vi "Calibration.vi"(7 "Show Front Panel":bool=TRUE, 8 "error in (no error)":errorcluster, 11 "Calibration File Path":path=path "C:/Program Files/GE/Dryer Performance Test/CalibrationDates.txt") -> (0 "error out":errorcluster, 3 "Calibration Data":string[][](array[string]))   [LabVIEW 2018]
uses:
  Type Definitions/Calibration.ctl
  Type Definitions/Calibration Time.ctl
  Type Definitions/Calibration SN.ctl
  Calibration Equipment.vi
  <vilib>/Utility/file.llb/Write Delimited Spreadsheet (string).vi
panel:
  out "concatenated string":string
  in  "Size":i32
  out "snta":string[](array[string])
  in  "Tab Control":enum32{"Calibration Dates", "Export Data"}(tab)
  in  "Equipment Description":T1
  in  "Manufacturer":T1
  in  "Model Number":T1
  in  "Calibration ID":T1
  in  "Complete":bool
  in  "Serial Number":T2
  in  "Last Calibrated":T3 {"Eq20" format="%<%x>T"; "Eq19" format="%<%x>T"; "Eq18" format="%<%x>T"; "Eq17" format="%<%x>T"; "Eq16" format="%<%x>T"; "Eq15" format="%<%x>T"; "Eq14" format="%<%x>T"; "Eq13" format="%<%x>T"; "Eq12" format="%<%x>T"; "Eq11" format="%<%x>T"; "Eq10" format="%<%x>T"; "Eq9" format="%<%x>T"; "Eq8" format="%<%x>T"; "Eq7" format="%<%x>T"; "Eq6" format="%<%x>T"; "Eq5" format="%<%x>T"; "Eq4" format="%<%x>T"; "Eq3" format="%<%x>T"; "Eq2" format="%<%x>T"; "Eq1" format="%<%x>T"}
  in  "Calibration Due":T3 {"Eq20" format="%<%x>T"; "Eq19" format="%<%x>T"; "Eq18" format="%<%x>T"; "Eq17" format="%<%x>T"; "Eq16" format="%<%x>T"; "Eq15" format="%<%x>T"; "Eq14" format="%<%x>T"; "Eq13" format="%<%x>T"; "Eq12" format="%<%x>T"; "Eq11" format="%<%x>T"; "Eq10" format="%<%x>T"; "Eq9" format="%<%x>T"; "Eq8" format="%<%x>T"; "Eq7" format="%<%x>T"; "Eq6" format="%<%x>T"; "Eq5" format="%<%x>T"; "Eq4" format="%<%x>T"; "Eq3" format="%<%x>T"; "Eq2" format="%<%x>T"; "Eq1" format="%<%x>T"}
  in  "Update":bool
  # "To Export Data: Right Click -> Export"
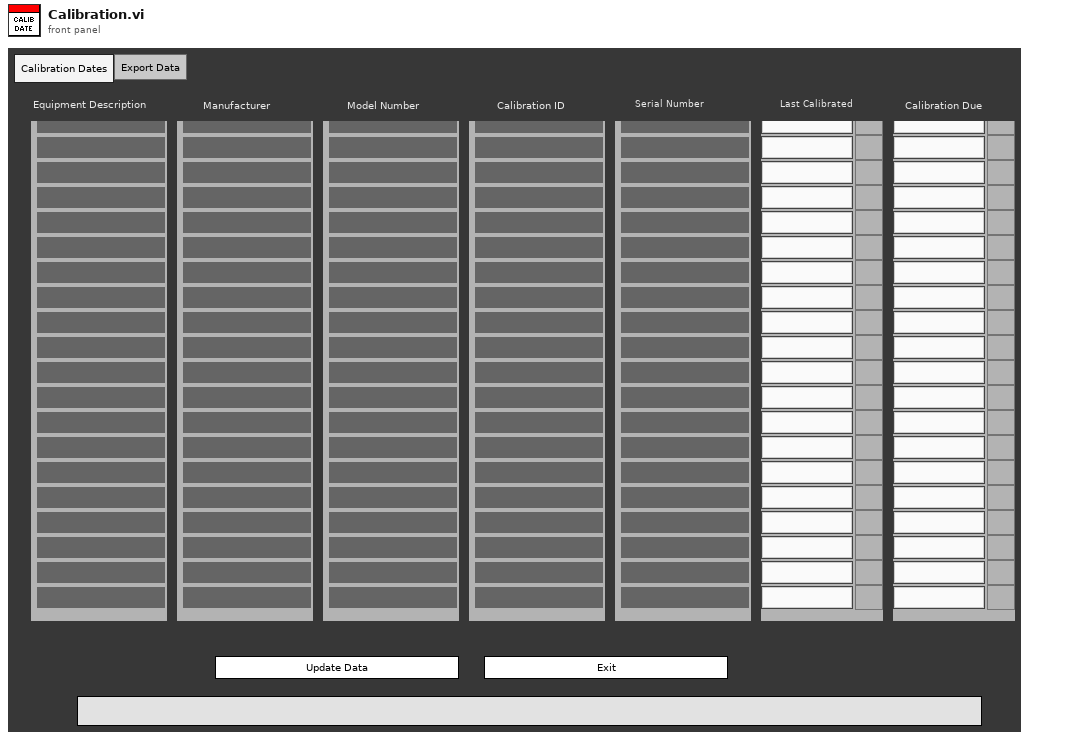
[diagram p1: front panel]
types:
  T1 = typedef "Calibration.ctl" = cluster{"Eq 1":string, "Eq 2":string, "Eq 3":string, "Eq 4":string, "Eq 5":string, "Eq 6":string, "Eq 7":string, "Eq 8":string, "Eq 9":string, "Eq 10":string, "Eq 11":string, "Eq 12":string, "Eq 13":string, "Eq 14":string, "Eq 15":string, "Eq 16":string, "Eq 17":string, "Eq 18":string, "Eq 19":string, "Eq 20":string}
  T2 = typedef "Calibration SN.ctl" = cluster{"Eq 1":string, "Eq 2":string, "Eq 3":string, "Eq 4":string, "Eq 5":string, "Eq 6":string, "Eq 7":string, "Eq 8":string, "Eq 9":string, "Eq 10":string, "Eq 11":string, "Eq 12":string, "Eq 13":string, "Eq 14":string, "Eq 15":string, "Eq 16":string, "Eq 17":string, "Eq 18":string, "Eq 19":string, "Eq 20":string}
  T3 = typedef "Calibration Time.ctl" = cluster{"Eq1":timestamp, "Eq2":timestamp, "Eq3":timestamp, "Eq4":timestamp, "Eq5":timestamp, "Eq6":timestamp, "Eq7":timestamp, "Eq8":timestamp, "Eq9":timestamp, "Eq10":timestamp, "Eq11":timestamp, "Eq12":timestamp, "Eq13":timestamp, "Eq14":timestamp, "Eq15":timestamp, "Eq16":timestamp, "Eq17":timestamp, "Eq18":timestamp, "Eq19":timestamp, "Eq20":timestamp}
  T4 = cluster{"Calibration Due":T3, "Last Calibrated":T3, "Serial Number":T2, "Calibration ID":T1, "Model Number":T1, "Manufacturer":T1, "Equipment Description":T1, "Size":i32}
  T5 = enum32{"invalid app kind", "Development System", "Run Time System", "Student Edition", "Embedded LabVIEW", "Evaluation", "Custom"}
  T6 = cluster{"Current VI Reference":refnum<vi>, "Close Panel on Exit?":bool}
  T7 = enum32{"Invalid", "Standard", "Closed", "Hidden", "Minimized", "Maximized"}
  T8 = cluster{"Core":cluster{"Current VI Reference":refnum<vi>, "Close Panel on Exit?":bool}, "Calibration Due":T3, "Calibration File Path":path, "Serial Number":T2, "Calibration ID":T1, "Total Array":string[][], "Size":i32, "Last Calibrated":T3, "Model Number":T1, "Manufacturer":T1, "Equipment Description":T1}
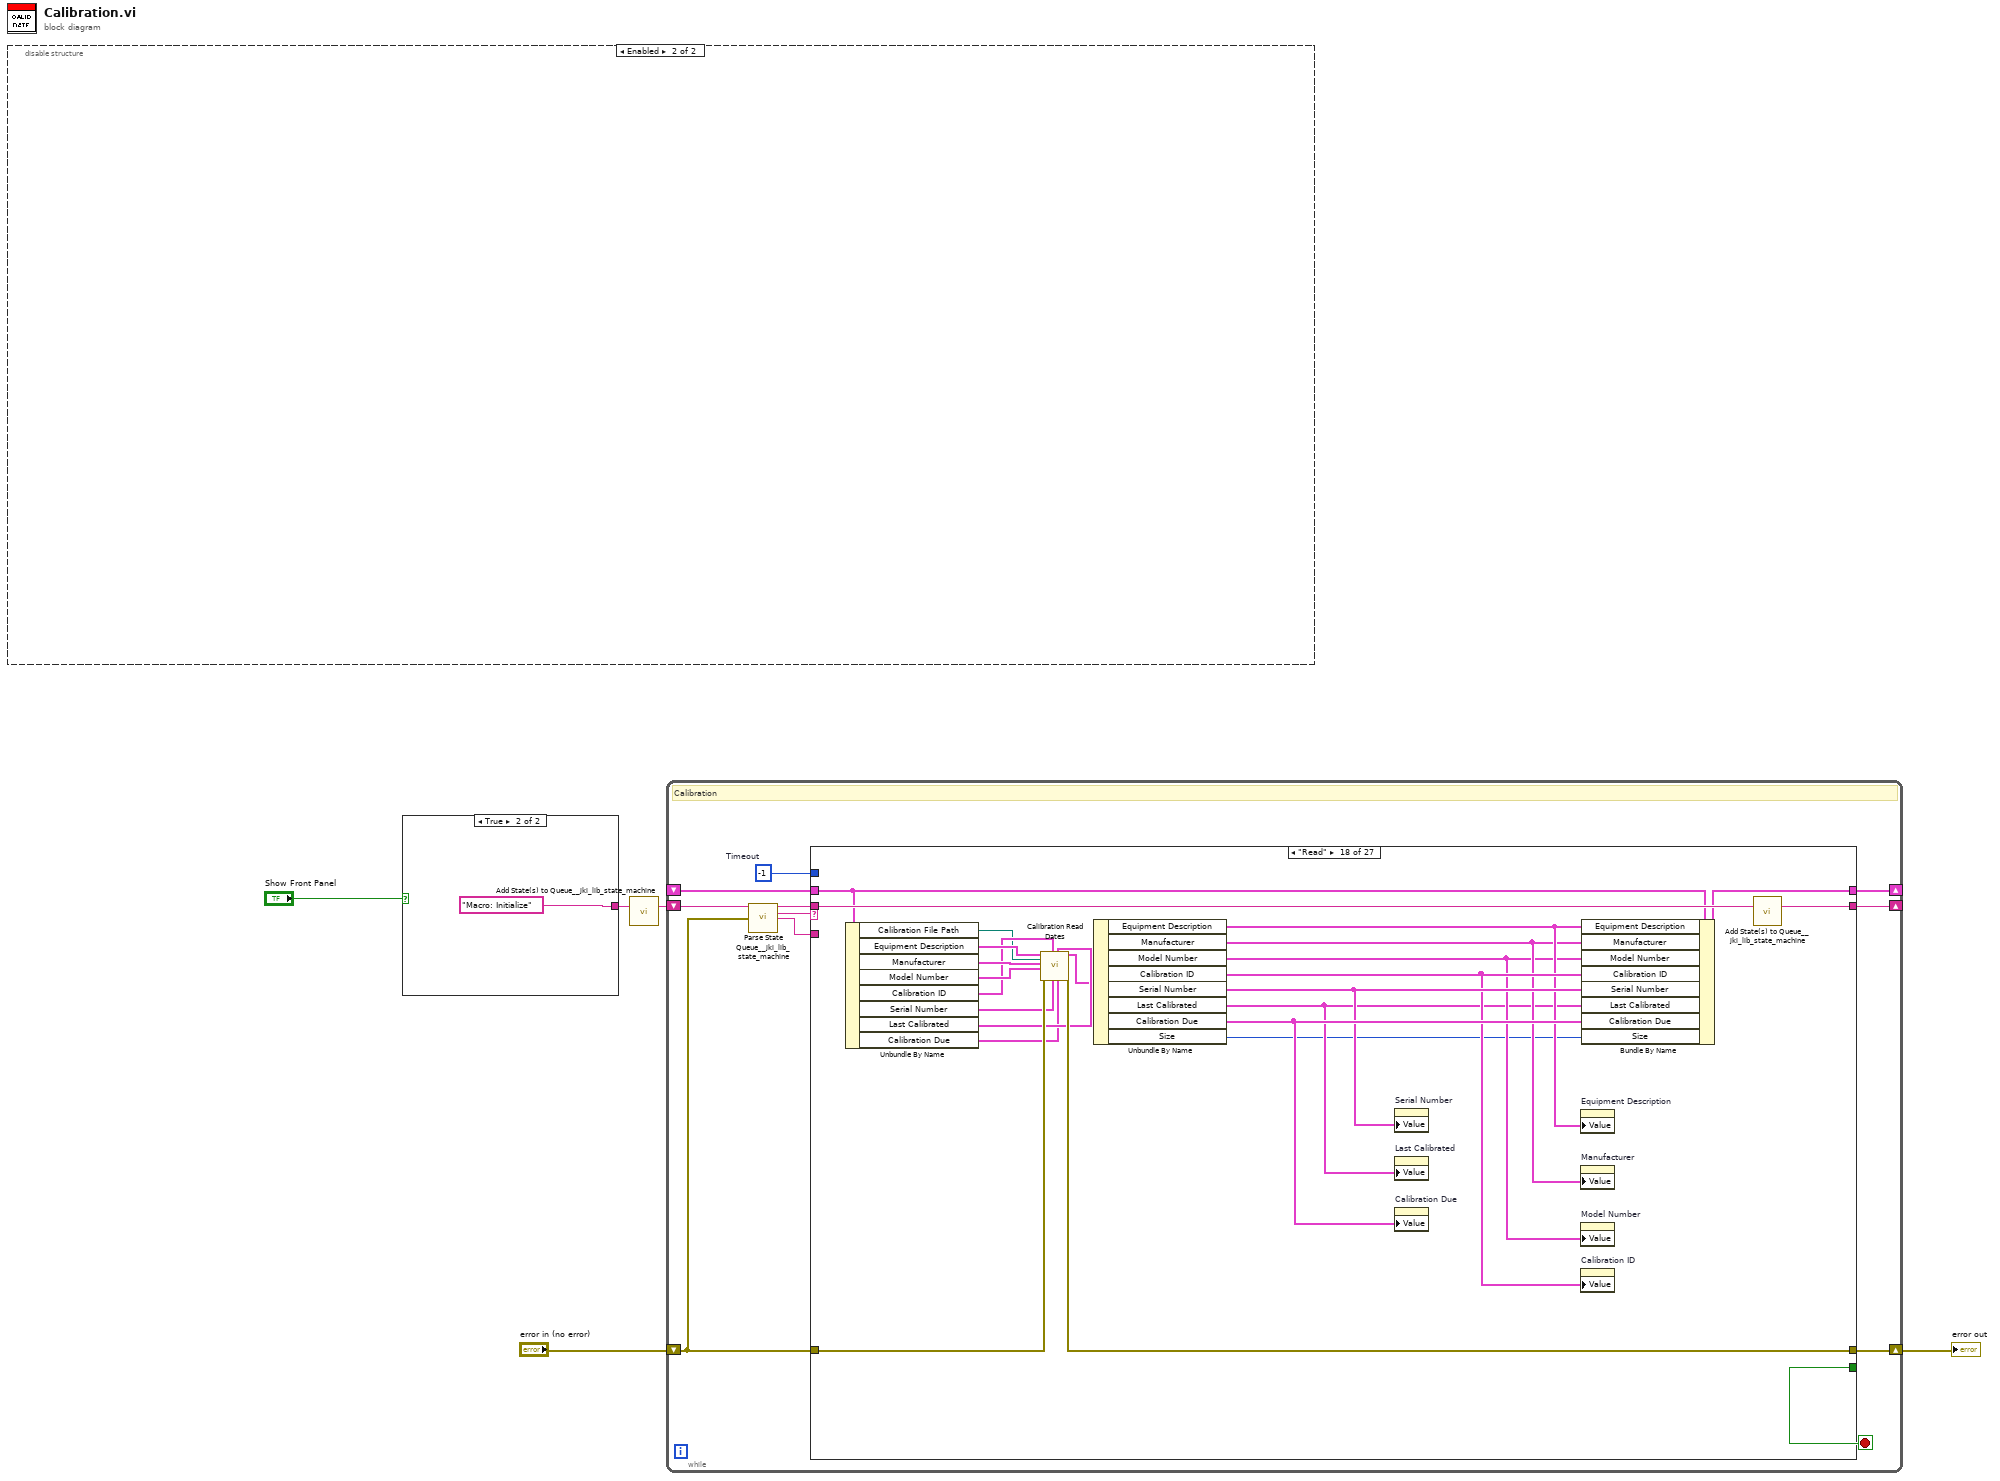
[diagram p0: block diagram]
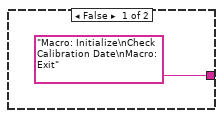
[diagram p2: hidden frame]
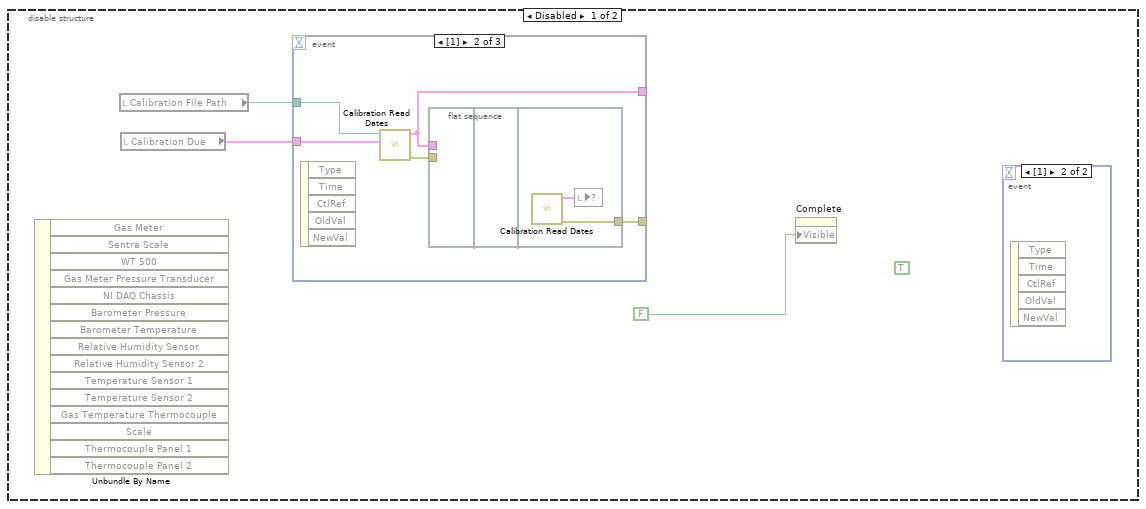
[diagram p3: hidden frame]
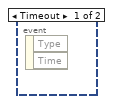
[diagram p4: hidden frame]
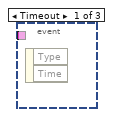
[diagram p5: hidden frame]
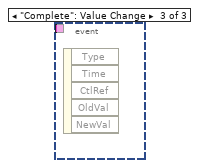
[diagram p6: hidden frame]
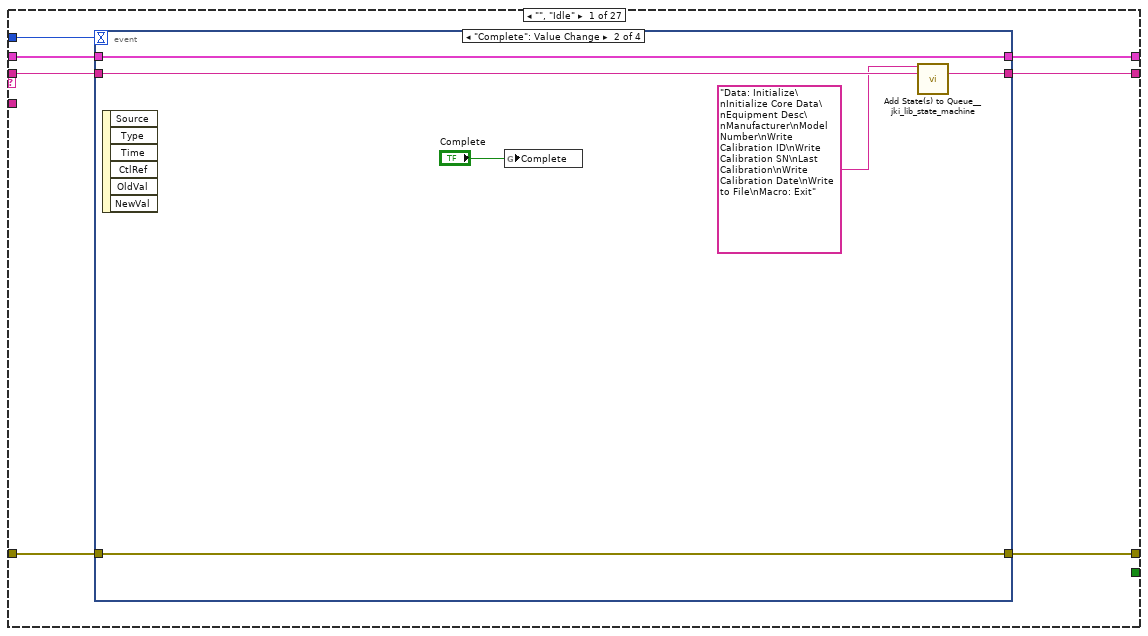
[diagram p7: hidden frame]
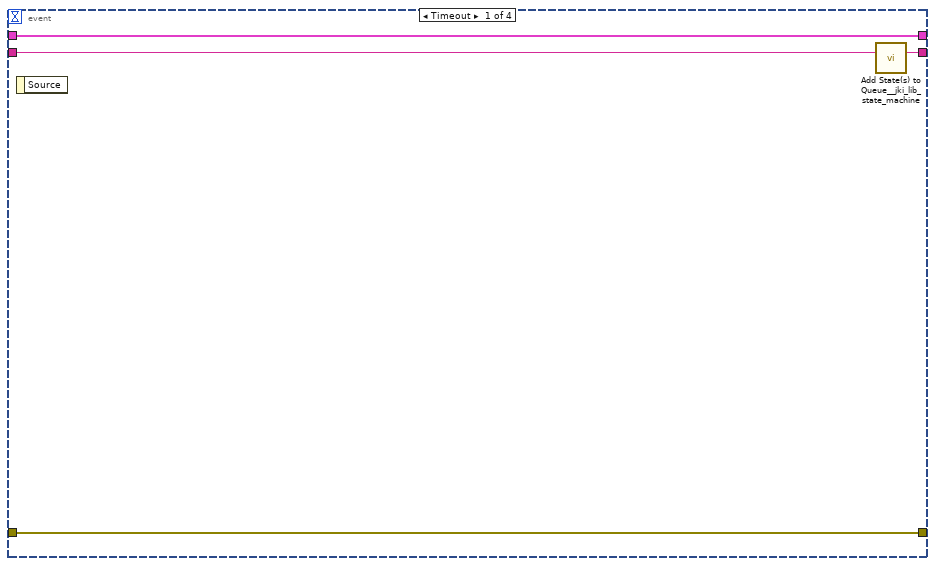
[diagram p8: hidden frame]
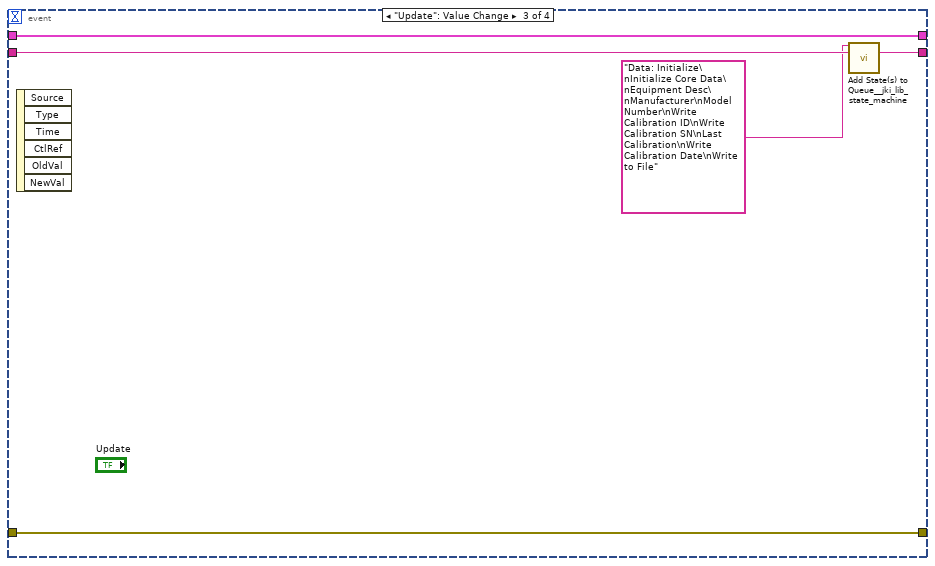
[diagram p9: hidden frame]
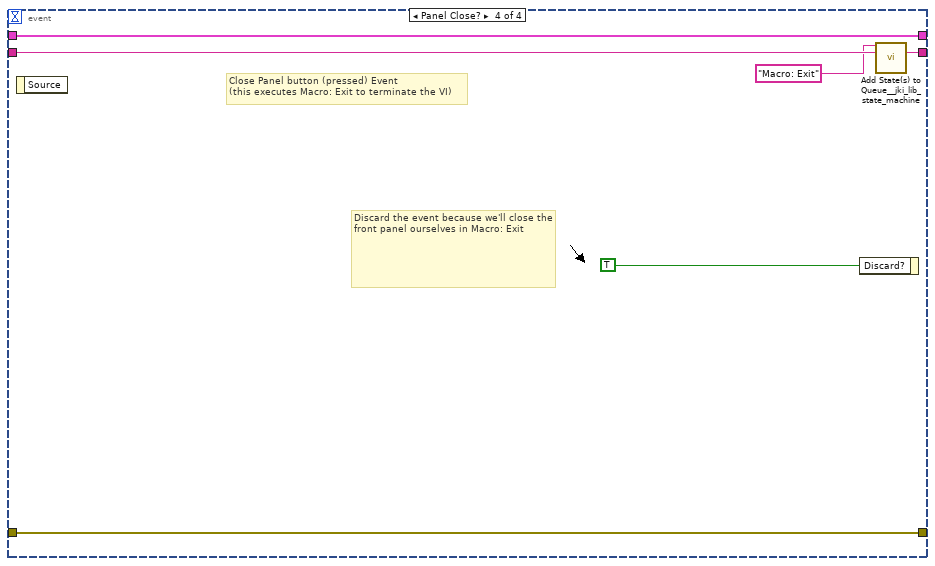
[diagram p10: hidden frame]
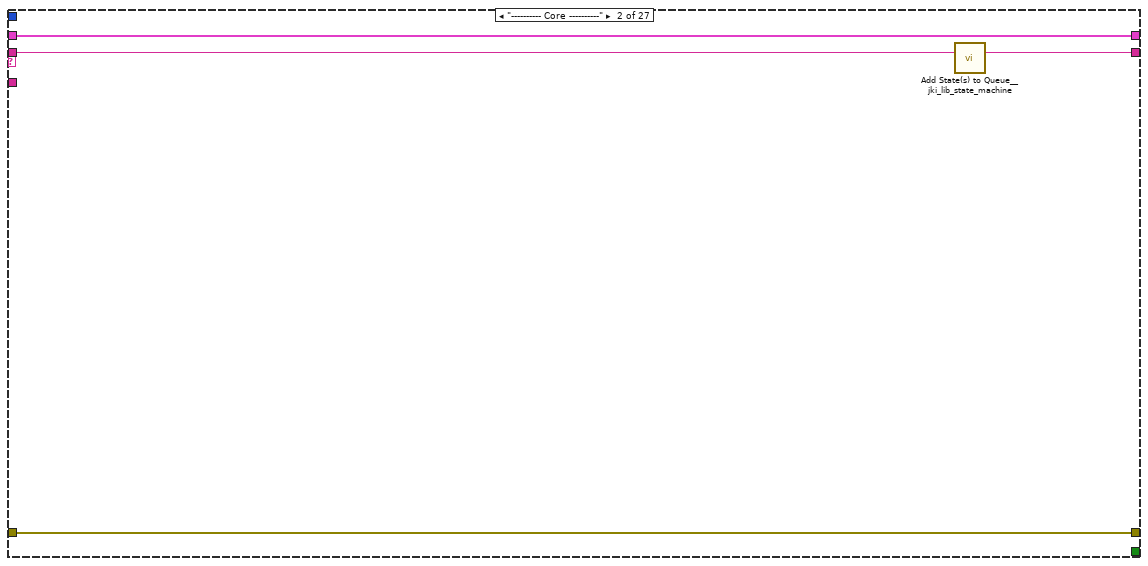
[diagram p11: hidden frame]
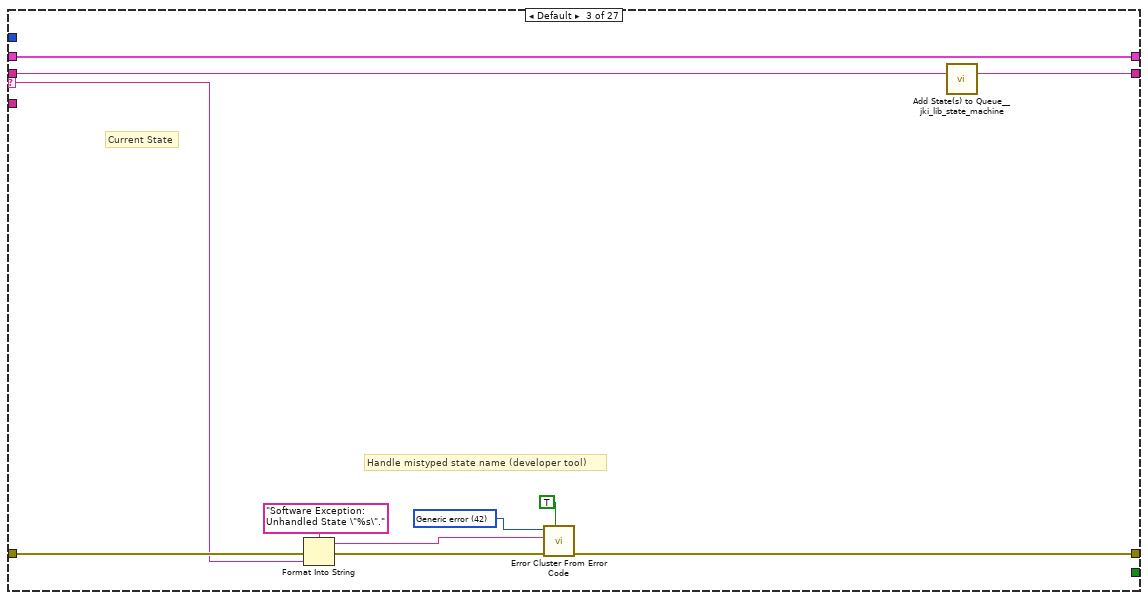
[diagram p12: hidden frame]
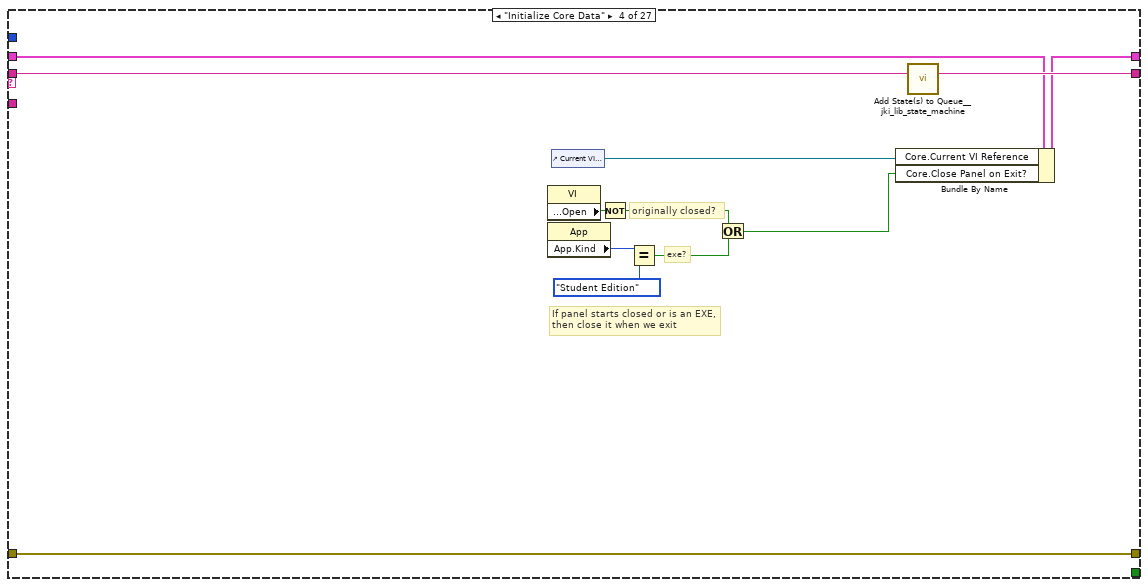
[diagram p13: hidden frame]
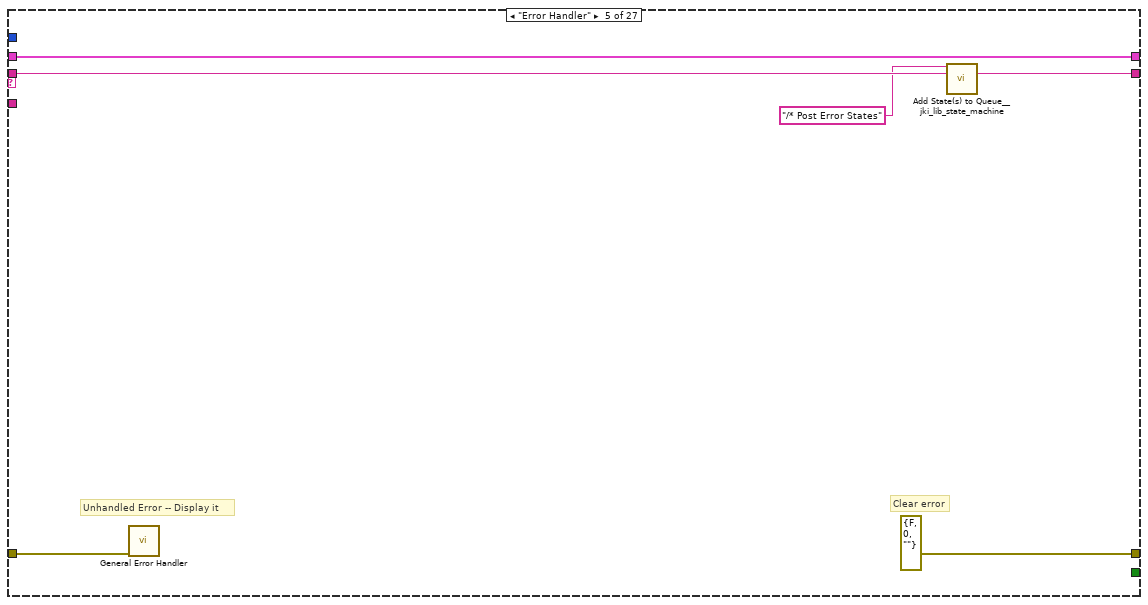
[diagram p14: hidden frame]
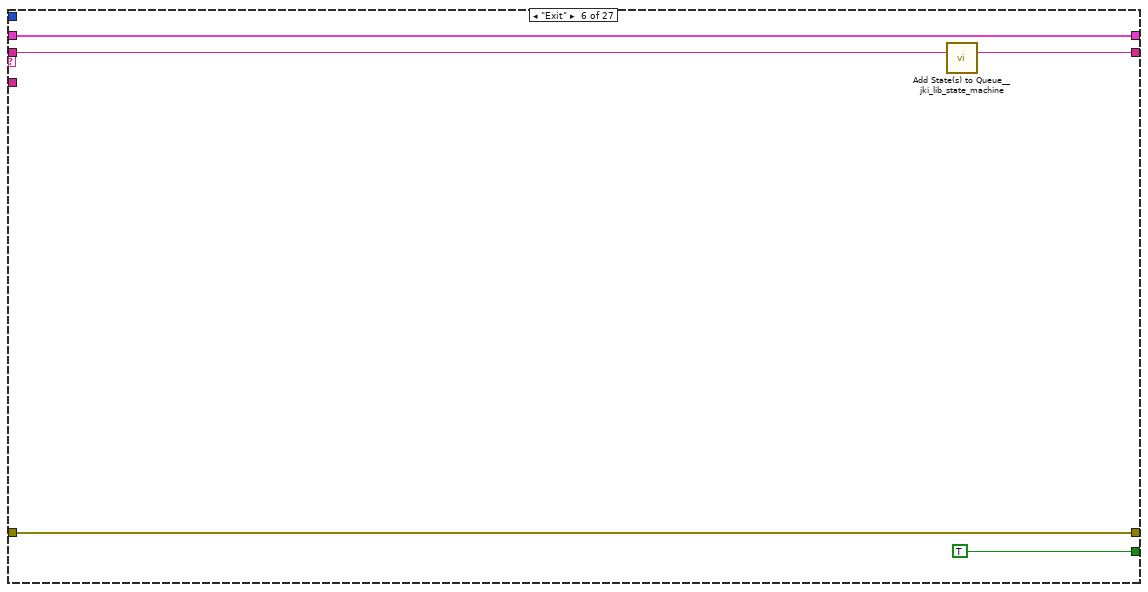
[diagram p15: hidden frame]
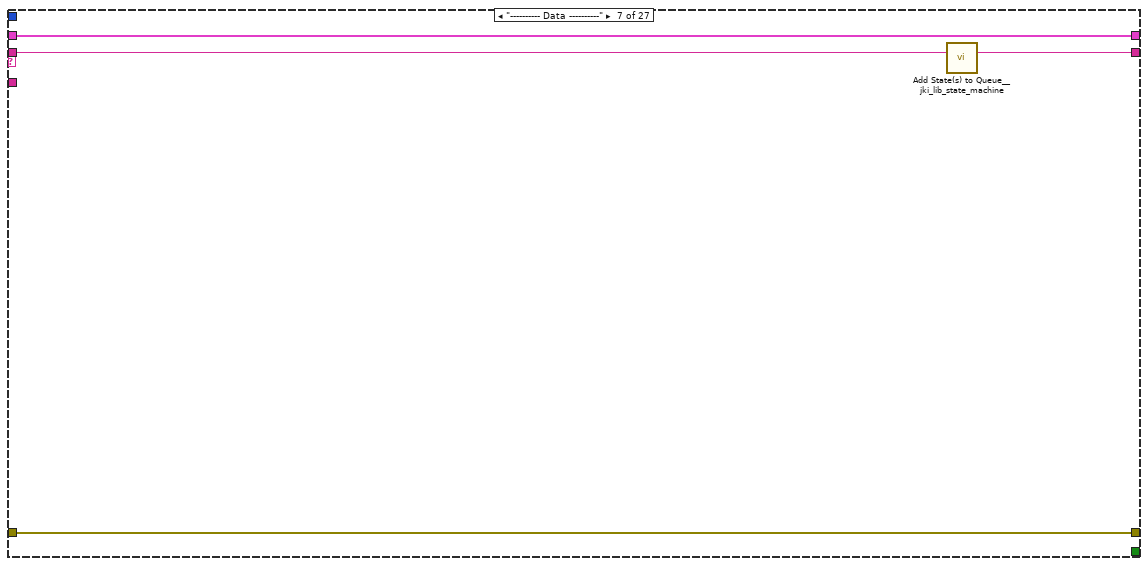
[diagram p16: hidden frame]
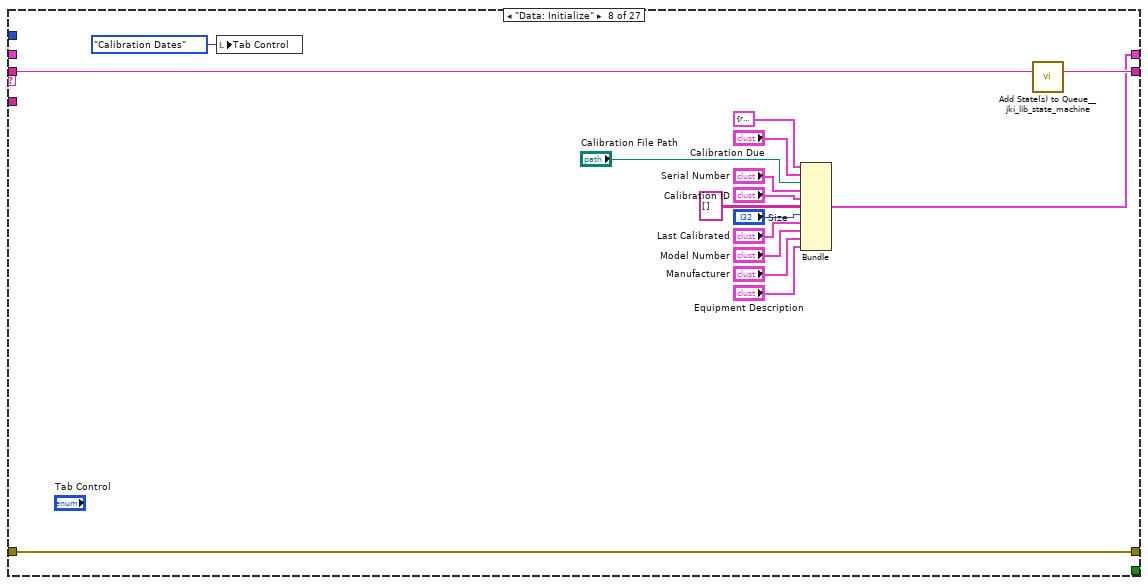
[diagram p17: hidden frame]
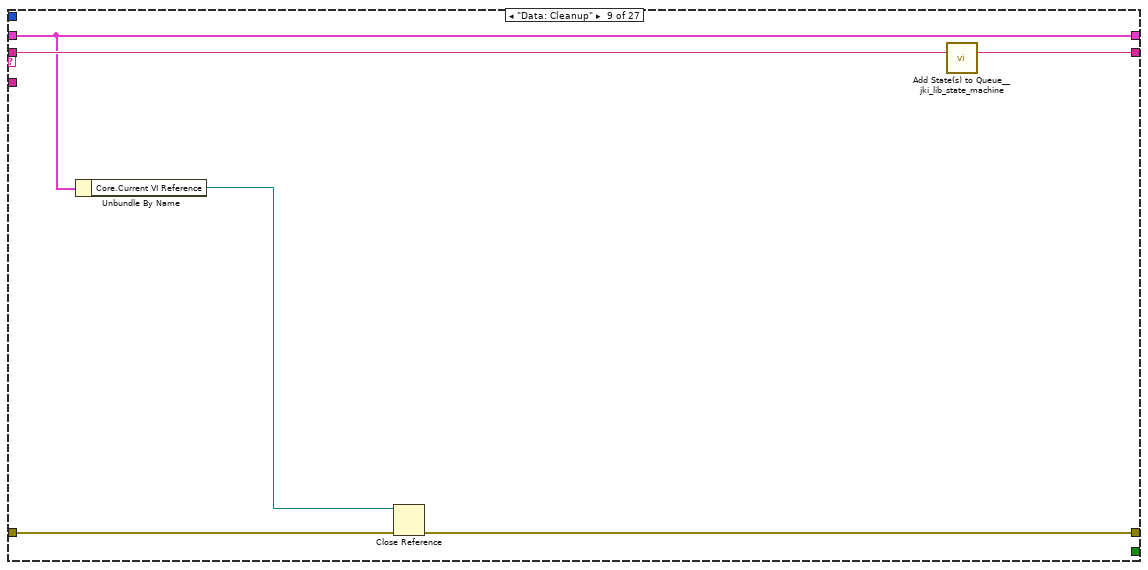
[diagram p18: hidden frame]
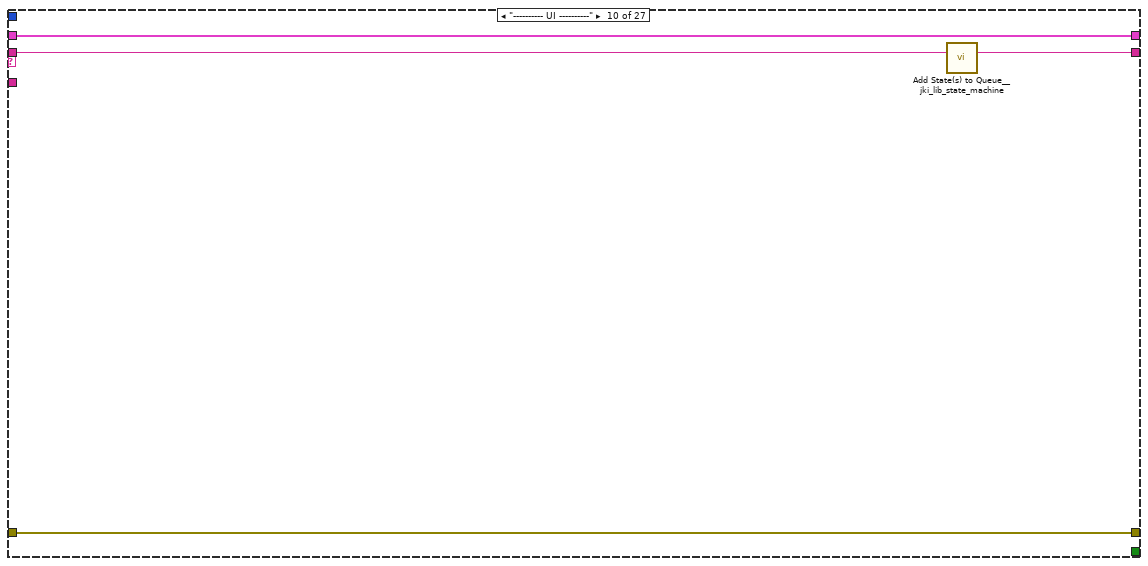
[diagram p19: hidden frame]
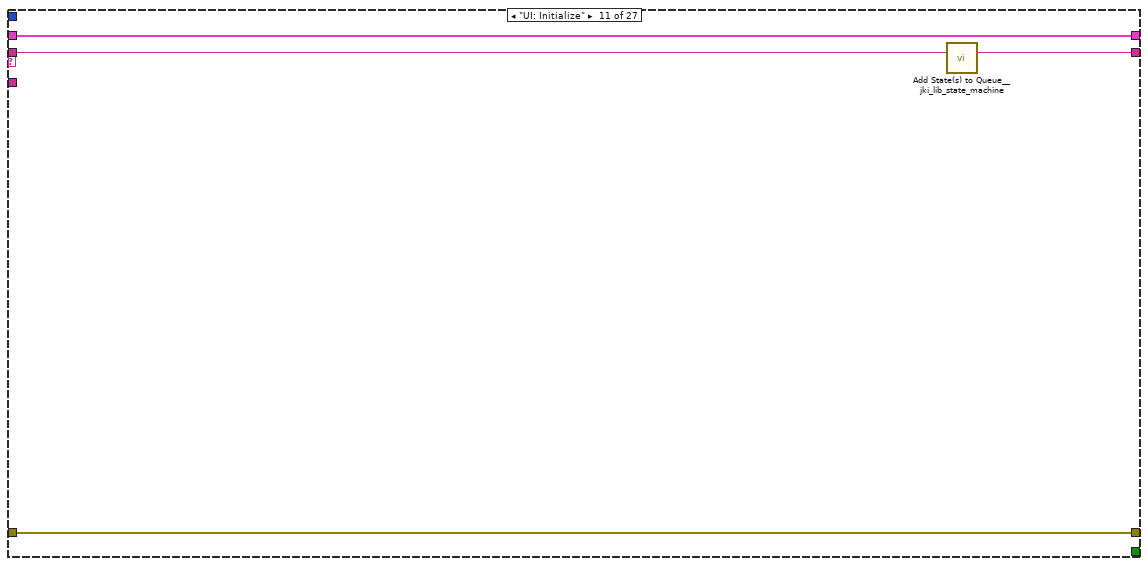
[diagram p20: hidden frame]
diagram:
  n1 = disable-structure shown="Enabled" {
    frame Disabled {
      w8 = TRUE ("Visible")
      n2 = Unbundle By Name() -> ()  [unwired: 1 in, 15 out]
      n3 = local read "Calibration File Path"() -> (w6:path)
      n4 = local read "Calibration Due"() -> (w7:T3)
      n5 = event shown="[1]" {
        selector: _ -> [_ _ _]
        dyn-events: _ -> [_ _ _]
        timeout: _ -> [_ _ _]
        tunnel: [_ w12 _] -> _
        tunnel: [_ w15 _] -> _
        tunnel: w7 -> [_ w14 _]
        tunnel: w6 -> [_ w13 _]
        event Timeout {
          n6 = event-data() -> ()  [unwired: 1 in, 2 out]
        }
        event #1 (no event record) {
          n7 = event-data() -> ()  [unwired: 1 in, 5 out]
          n8 = call "Calibration Read Dates.vi"("Manufacturer"=w14, "Equipment Description"=w13) -> ("error out"=w11:errorcluster, "output cluster"=w12:T4)  [unwired: 8 in]
          n9 = flat-sequence {
            tunnel: w11 -> [_]
            tunnel: w12 -> [_]
            tunnel: [w16] -> w15
            frame #0 {
            }
            frame #1 {
            }
            frame #2 {
              n10 = call "Calibration Read Dates.vi"() -> ("error out"=w16:errorcluster, "output cluster"=w17:T4)  [unwired: 10 in]
              n11 = local write item#-1(w17) -> ()
            }
          }
        }
        event "Complete": Value Change {
          n12 = event-data() -> ()  [unwired: 1 in, 5 out]
        }
      }
      n13 = property on="Complete" class="Bool"("Visible"=FALSE) -> (error out=w9:errorcluster)  [unwired: 2 in, 1 out]
      n14 = event shown="[1]" {
        selector: _ -> [_ _]
        dyn-events: _ -> [_ _]
        timeout: _ -> [_ _]
        event Timeout {
          n15 = event-data() -> ()  [unwired: 1 in, 2 out]
        }
        event #1 (no event record) {
          n16 = event-data() -> ()  [unwired: 1 in, 5 out]
        }
      }
    }
    frame Enabled {
    }
  }
  n17 = case shown="True" "Show Front Panel" {
    tunnel: ["Macro: Initialize\nCheck Calibration Date\nMacro: Exit" "Macro: Initialize"] -> w4
    frame False {
    }
    frame True {
    }
  }
  n18 = call <vilib>:"Add State(s) to Queue__jki_lib_state_machine.vi"("State(s) in (\"\")"=w4) -> ("States Out"=w5:string)  [unwired: 14 in]
  n19 = while "Cailbration" {
    shift-right: [w23] -> _
    shift-left: _ -> [w22]
    shift-right: [w26] -> w2
    shift-left: "error in (no error)" -> [w20]
    shift-right: [w25] -> _
    shift-left: w5 -> [w27]
    stop <- w24 stop-if-true
    w21 = -1  # Timeout
    # "Calibration"
    n20 = call <vilib>:"Parse State Queue__jki_lib_state_machine.vi"("State Queue"=w27, "Error In (no error)"=w20) -> ("Remaining States"=w29:string, "Current State"=w30:string, "Arguments"=w28:string)  [unwired: 11 in]
    n21 = case shown="\"Read\"" w30 {
      selector: w30 -> [_ _ w63 _ _ _ _ _ _ _ _ _ _ _ _ _ _ _ _ _ _ _ _ _ _ _ _]
      tunnel: w29 -> [w37 w62 w67 w85 w91 w96 w100 w116 w122 w126 w130 w136 w147 w173 w178 w188 w192 w215 w227 w369 w429 w489 w549 w609 w669 w751 w830]
      tunnel: w28 -> [_ _ _ _ _ _ _ _ _ _ _ w131 w141 _ _ _ _ _ _ _ _ _ _ _ _ _ _]
      tunnel: w22 -> [w35 w59 w65 w76 w88 w94 w97 _ w117 w123 w128 w134 w143 w170 w175 w185 w189 w213 w225 w363 w423 w483 w543 w603 w662 w744 w828]
      tunnel: [w34 w60 w69 w82 errorcluster {"status"=FALSE, "code"=0, "source"=""} ("error out") w93 w98 w113 w118 w124 w127 w132 w144 w171 w176 w186 w190 w210 w224 w364 w424 w484 w544 w604 w664 w746 w825] -> w26
      tunnel: w20 -> [w33 w60 w68 w82 w87 w93 w98 w113 w119 w124 w127 w133 w145 w171 w176 w186 w190 w211 w224 w365 w425 w485 w545 w605 w665 w747 w825]
      tunnel: [w36 w61 w66 w84 w90 w95 w99 w115 w121 w125 w129 w135 w146 w172 w177 w187 w191 w214 w226 w368 w428 w488 w548 w608 w668 w750 w829] -> w25
      tunnel: [_ _ _ _ _ TRUE _ _ _ _ _ _ _ _ _ _ _ _ _ _ _ _ _ _ _ _ _] -> w24
      tunnel: [w32 w59 w65 w83 w88 w94 w97 w114 w117 w123 w128 w134 w143 w170 w175 w185 w189 w212 w225 w362 w422 w482 w542 w602 w661 w743 w828] -> w23
      tunnel: w21 -> [w31 _ _ _ _ _ _ _ _ _ _ _ _ _ _ _ _ _ _ _ _ _ _ _ _ _ _]
      frame "", "Idle" {
        n22 = event shown="[1] \"Complete\": Value Change" {
          selector: _ -> [_ _ _ _]
          dyn-events: _ -> [_ _ _ _]
          timeout: w31 -> [_ _ _ _]
          tunnel: w37 -> [w41 w46 w50 w58]
          tunnel: [w40 w47 w49 w57] -> w36
          tunnel: w35 -> [w38 w43 w51 w55]
          tunnel: [w39 w45 w52 w56] -> w34
          tunnel: w33 -> [w39 w45 w52 w56]
          tunnel: [w38 w43 w51 w55] -> w32
          event Timeout {
            n23 = event-data() -> ()  [unwired: 1 in, 1 out]
            n24 = call <vilib>:"Add State(s) to Queue__jki_lib_state_machine.vi"("State(s) in (\"\")"=w41) -> ("States Out"=w40:string)  [unwired: 14 in]
          }
          event "Complete": Value Change {
            n25 = event-data() -> ()  [unwired: 1 in, 6 out]
            n26 = global write "Calibration Equipment.vi" "Complete"("Complete") -> ()
            n27 = call <vilib>:"Add State(s) to Queue__jki_lib_state_machine.vi"("State(s) in Front (\"\")"="Data: Initialize\nInitialize Core Data\nEquipment Desc\nManufacturer\nModel Number\nWrite Calibration ID\nWrite Calibration SN\nLast Calibration\nWrite Calibration Date\nWrite to File\nMacro: Exit", "State(s) in (\"\")"=w46) -> ("States Out"=w47:string)  [unwired: 13 in]
          }
          event "Update": Value Change {
            n28 = event-data() -> ()  [unwired: 1 in, 6 out]
            n29 = call <vilib>:"Add State(s) to Queue__jki_lib_state_machine.vi"("State(s) in Front (\"\")"="Data: Initialize\nInitialize Core Data\nEquipment Desc\nManufacturer\nModel Number\nWrite Calibration ID\nWrite Calibration SN\nLast Calibration\nWrite Calibration Date\nWrite to File", "State(s) in (\"\")"=w50) -> ("States Out"=w49:string)  [unwired: 13 in]
          }
          event Panel Close? {
            # "Discard the event because we'll close the front panel ourselves in Macro: Exit"
            # "Close Panel button (pressed) Event\n(this executes Macro: Exit to terminate the VI)"
            n30 = event-data() -> ()  [unwired: 1 in, 1 out]
            n31 = event-data("Discard?"=TRUE) -> ()  [unwired: 1 in, 1 out]
            n32 = call <vilib>:"Add State(s) to Queue__jki_lib_state_machine.vi"("State(s) in Front (\"\")"="Macro: Exit", "State(s) in (\"\")"=w58) -> ("States Out"=w57:string)  [unwired: 13 in]
          }
        }
      }
      frame "---------- Core ----------" {
        n33 = call <vilib>:"Add State(s) to Queue__jki_lib_state_machine.vi"("State(s) in (\"\")"=w62) -> ("States Out"=w61:string)  [unwired: 14 in]
      }
      frame Default {
        w72 = 42 items=["No error", "Argument error", "Memory is full", "Out of zone", "End of file", "File already open", "Generic file I/O error", "File not found", "File permission error", "Disk is full", "Duplicate path", "Too many files open", "System feature not enabled", "Resource file not found", "Cannot add resource", "Resource not found", "Image not found", "Image memory error", "Pen does not exist", "Config type invalid", "Config token not found", "Config parse error", "Config memory error", "Bad external code format", "Bad external code offset", "External code not present", "Null window", "Destroy window error", "Null menu", "Print aborted", "Bad print record", "Print driver error", "Windows error during printing", "Memory error during printing", "Print dialog error", "Generic print error", "Invalid device refnum", "Device not found", "Device parameter error", "Device unit error", "Cannot open device", "Device call aborted", "Generic error", "Cancelled by user", "Object ID too low", "Object ID too high", "Object not in heap", "Unknown heap", "Unknown object (invalid DefProc)", "Unknown object (DefProc not in table)", "Message out of range", "Invalid (null) method", "Unknown message", "Manager call not supported", "Bad address", "Network operation in progress", "Network operation timed out", "Connection is busy", "Network attribute not supported", "Network error", "Address in use", "System out of memory", "Connection aborted", "Connection refused", "Not connected", "Already connected", "Connection closed", "Initialization error (interapplication manager)", "Bad occurrence", "Wait on unbound occurrence handler", "Occurrence queue overflow", "Datalog type conflict", "Unused", "Unrecognized type (interapplication manager)", "Memory corrupt", "Failed to make temporary DLL", "Old CIN version", "Drag socket not found", "Failed to load drop-object", "Failed to register OLE object", "Failed to release OLE object", "Format specifier type mismatch", "Unknown format specifier", "Too few format specifiers", "Too many format specifiers", "Scan failed", "Newer CIN version", "Error converting to variant", "Runtime menu error", "Password tampered", "Variant attribute not found", "Incompatible variant data type", "Event data is not available", "Event Store is not present", "Occurrence is not found", "Event Queue is not created", "Event info is not available", "Refnum passed is NULL", "Error retrieving Class GUID", "Error retrieving CoClass GUID", "Error retrieving TypeLib GUID.", "Bad built application magic bytes.", "Specific driver is different from the specific driver associated with the Logical Name.", "There is no session opened to the class driver.", "Max Error", "MAX - Error with config objects", "MAX - Error loading configuration", "MAX - Group not supported"]
        # "Current State"
        # "Handle mistyped state name (developer tool)"
        n34 = Format Into String(format string="Software Exception: Unhandled State \"%s\"." ("message"), error in=w68, w63) -> (resulting string=w71:string, error out=w70:errorcluster)  [unwired: 1 in]
        n35 = call <vilib>:"Error Cluster From Error Code.vi"("show call chain? (False)"=TRUE, "error in (no error)"=w70, "error message (\"\")"=w71, "error code (0)"=w72) -> ("error out"=w69:errorcluster)  [unwired: 5 in]
        n36 = call <vilib>:"Add State(s) to Queue__jki_lib_state_machine.vi"("State(s) in (\"\")"=w67) -> ("States Out"=w66:string)  [unwired: 14 in]
      }
      frame "Initialize Core Data" {
        # "originally closed?"
        # "exe?"
        # "If panel starts closed or is an EXE, then close it when we exit"
        n37 = property class="VI"() -> ("Front Panel.Open"=w81:bool)  [unwired: 2 in, 2 out]
        n38 = property class="App"() -> ("App.Kind"=w80:T5)  [unwired: 2 in, 2 out]
        n39 = control-ref of="Current VI Reference"() -> (w74:refnum<vi>)
        n40 = Not(x=w81) -> (.not. x?=w78:bool)
        n41 = Equal?(x=w80, y=T5."Student Edition" ("Application:Kind")) -> (x = y?=w77:bool)
        n42 = Or(x=w78, y=w77) -> (x .or. y?=w75:bool)
        n43 = Bundle By Name(cluster=w76, "Core.Current VI Reference"=w74, "Core.Close Panel on Exit?"=w75) -> (w83:T8)
        n44 = call <vilib>:"Add State(s) to Queue__jki_lib_state_machine.vi"("State(s) in (\"\")"=w85) -> ("States Out"=w84:string)  [unwired: 14 in]
      }
      frame "Error Handler" {
        # "Unhandled Error -- Display it"
        # "Clear error"
        n45 = call <vilib>:"General Error Handler.vi"("error in (no error)"=w87) -> ()  [unwired: 10 in, 5 out]
        n46 = call <vilib>:"Add State(s) to Queue__jki_lib_state_machine.vi"("State(s) in Front (\"\")"="/* Post Error States", "State(s) in (\"\")"=w91) -> ("States Out"=w90:string)  [unwired: 13 in]
      }
      frame "Exit" {
        n47 = call <vilib>:"Add State(s) to Queue__jki_lib_state_machine.vi"("State(s) in (\"\")"=w96) -> ("States Out"=w95:string)  [unwired: 14 in]
      }
      frame "---------- Data ----------" {
        n48 = call <vilib>:"Add State(s) to Queue__jki_lib_state_machine.vi"("State(s) in (\"\")"=w100) -> ("States Out"=w99:string)  [unwired: 14 in]
      }
      frame "Data: Initialize" {
        n49 = local write "Tab Control"(enum32{"Calibration Dates", "Export Data"}."Calibration Dates" ("Tab Control")) -> ()
        n50 = Bundle("Core"=T6 {"Current VI Reference"=refnum, "Close Panel on Exit?"=TRUE}, "Calibration Due"="Calibration Due", "Calibration File Path"="Calibration File Path", "Serial Number"="Serial Number", "Calibration ID"="Calibration ID", "Total Array"=string[][] [], "Size"="Size", "Last Calibrated"="Last Calibrated", "Model Number"="Model Number", "Manufacturer"="Manufacturer", "Equipment Description"="Equipment Description") -> (w114:T8)  [unwired: 1 in]
        n51 = call <vilib>:"Add State(s) to Queue__jki_lib_state_machine.vi"("State(s) in (\"\")"=w116) -> ("States Out"=w115:string)  [unwired: 14 in]
      }
      frame "Data: Cleanup" {
        n52 = Unbundle By Name(w117) -> ("Core.Current VI Reference"=w120:refnum<vi>)
        n53 = Close Reference(reference=w120, error in (no error)=w119) -> (error out=w118:errorcluster)
        n54 = call <vilib>:"Add State(s) to Queue__jki_lib_state_machine.vi"("State(s) in (\"\")"=w122) -> ("States Out"=w121:string)  [unwired: 14 in]
      }
      frame "---------- UI ----------" {
        n55 = call <vilib>:"Add State(s) to Queue__jki_lib_state_machine.vi"("State(s) in (\"\")"=w126) -> ("States Out"=w125:string)  [unwired: 14 in]
      }
      frame "UI: Initialize" {
        n56 = call <vilib>:"Add State(s) to Queue__jki_lib_state_machine.vi"("State(s) in (\"\")"=w130) -> ("States Out"=w129:string)  [unwired: 14 in]
      }
      frame "UI: Cursor Set" {
        # "Argument"
        n57 = case shown="\"Idle\", Default" w131 {
          tunnel: w133 -> [w138 w140]
          tunnel: [w137 w139] -> w132
          frame "Idle", Default {
            n58 = call <vilib>:"Unset Busy.vi"("error in (no error)"=w138) -> ("error out"=w137:errorcluster)  [unwired: 10 in]
          }
          frame "Busy" {
            n59 = call <vilib>:"Set Busy.vi"("error in (no error)"=w140) -> ("error out"=w139:errorcluster)  [unwired: 9 in, 1 out]
          }
        }
        n60 = call <vilib>:"Add State(s) to Queue__jki_lib_state_machine.vi"("State(s) in (\"\")"=w136) -> ("States Out"=w135:string)  [unwired: 14 in]
      }
      frame "UI: Front Panel State" {
        # "Argument"
        n61 = Unbundle By Name(w143) -> ("Core.Current VI Reference"=w142:refnum<vi>)
        n62 = case shown="\"Open\", Default" w141 {
          tunnel: w145 -> [w151 w164]
          tunnel: [w153 w165] -> w144
          tunnel: w142 -> [w152 w162]
          frame "Open", Default {
            n63 = property class="VI"(reference=w152, error in=w151) -> (reference out=w149:refnum<vi>, error out=w150:errorcluster, "Front Panel.Open"=w148:bool)
            n64 = case shown="True" w148 {
              tunnel: [w156 w159] -> w153
              tunnel: w150 -> [w155 w159]
              tunnel: w149 -> [w154 _]
              frame False {
                n65 = invoke class="VI" method="FP.Open"(reference=w154, error in=w155, "Activate"=TRUE, "State"=T7."Standard") -> (error out=w156:errorcluster)  [unwired: 1 in, 4 out]
              }
              frame True {
              }
            }
          }
          frame "Close" {
            n66 = property class="VI"(reference=w162, error in=w164) -> (reference out=w161:refnum<vi>, error out=w163:errorcluster, "Front Panel.Open"=w160:bool)
            n67 = case shown="True" w160 {
              tunnel: [w166 w169] -> w165
              tunnel: w163 -> [w166 w168]
              tunnel: w161 -> [_ w167]
              frame False {
              }
              frame True {
                n68 = invoke class="VI" method="FP.Close"(reference=w167, error in=w168) -> (error out=w169:errorcluster)  [unwired: 1 in, 2 out]
              }
            }
          }
        }
        n69 = call <vilib>:"Add State(s) to Queue__jki_lib_state_machine.vi"("State(s) in (\"\")"=w147) -> ("States Out"=w146:string)  [unwired: 14 in]
      }
      frame "---------- Macro ----------" {
        n70 = call <vilib>:"Add State(s) to Queue__jki_lib_state_machine.vi"("State(s) in (\"\")"=w173) -> ("States Out"=w172:string)  [unwired: 14 in]
      }
      frame "Macro: Initialize" {
        w174 = "Data: Initialize\nInitialize Core Data\nUI: Initialize\nUI: Front Panel State >> Open\nRead\nCheck Calibration Date"  # Data: Initialize Initialize Core Data UI: Initialize UI: Front Panel State >> Open Read Check Calibration Date
        n71 = call <vilib>:"Add State(s) to Queue__jki_lib_state_machine.vi"("State(s) in Front (\"\")"=w174, "State(s) in (\"\")"=w178) -> ("States Out"=w177:string)  [unwired: 13 in]
      }
      frame "Macro: Exit" {
        n72 = Unbundle By Name(w185) -> ("Core.Close Panel on Exit?"=w184:bool)
        n73 = Select(t="UI: Front Panel State >> Close", s=w184, f="") -> (s? t:f=w181:string)
        n74 = call <vilib>:"Add State(s) to Queue__jki_lib_state_machine.vi"("State(s) in (\"\")"=w181, "State(s) at Back (\"\")"="Data: Cleanup\nExit") -> ("States Out"=w179:string)  [unwired: 13 in]
        n75 = call <vilib>:"Add State(s) to Queue__jki_lib_state_machine.vi"("State(s) in Front (\"\")"=w179, "State(s) in (\"\")"=w188) -> ("States Out"=w187:string)  [unwired: 13 in]
      }
      frame "---------- New Category ----------" {
        n76 = call <vilib>:"Add State(s) to Queue__jki_lib_state_machine.vi"("State(s) in (\"\")"=w192) -> ("States Out"=w191:string)  [unwired: 14 in]
      }
      frame "Read" {
        n77 = Unbundle By Name(w213) -> ("Calibration File Path"=w202:path, "Equipment Description"=w209:T1, "Manufacturer"=w208:T1, "Model Number"=w207:T1, "Calibration ID"=w206:T1, "Serial Number"=w205:T2, "Last Calibrated"=w204:T3, "Calibration Due"=w203:T3)
        n78 = call "Calibration Read Dates.vi"("Equipment Description"=w209, "File Path"=w202, "Manufacturer"=w208, "Model Number"=w207, "error in (no error)"=w211, "Calibration ID"=w206, "Serial Number"=w205, "Last Calibrated"=w204, "Calibration Due"=w203) -> ("output cluster"=w201:T4, "error out"=w210:errorcluster)  [unwired: 9 in]
        n79 = Unbundle By Name(w201) -> ("Equipment Description"=w197:T1, "Manufacturer"=w196:T1, "Model Number"=w195:T1, "Calibration ID"=w198:T1, "Serial Number"=w199:T2, "Last Calibrated"=w194:T3, "Calibration Due"=w200:T3, "Size"=w193:i32)
        n80 = property on="Serial Number" class="Clust (strict)"("Value"=w199) -> ()  [unwired: 2 in, 2 out]
        n81 = property on="Last Calibrated" class="Clust (strict)"("Value"=w194) -> ()  [unwired: 2 in, 2 out]
        n82 = property on="Calibration Due" class="Clust (strict)"("Value"=w200) -> ()  [unwired: 2 in, 2 out]
        n83 = property on="Equipment Description" class="Clust (strict)"("Value"=w197) -> ()  [unwired: 2 in, 2 out]
        n84 = property on="Manufacturer" class="Clust (strict)"("Value"=w196) -> ()  [unwired: 2 in, 2 out]
        n85 = property on="Model Number" class="Clust (strict)"("Value"=w195) -> ()  [unwired: 2 in, 2 out]
        n86 = property on="Calibration ID" class="Clust (strict)"("Value"=w198) -> ()  [unwired: 2 in, 2 out]
        n87 = Bundle By Name(cluster=w213, "Equipment Description"=w197, "Manufacturer"=w196, "Model Number"=w195, "Calibration ID"=w198, "Serial Number"=w199, "Last Calibrated"=w194, "Calibration Due"=w200, "Size"=w193) -> (w212:T8)
        n88 = call <vilib>:"Add State(s) to Queue__jki_lib_state_machine.vi"("State(s) in (\"\")"=w215) -> ("States Out"=w214:string)  [unwired: 14 in]
      }
      frame "Check Calibration Date" {
        n89 = Unbundle By Name(w225) -> ("Size"=w223:i32, "Calibration Due"=w217:T3)
        n90 = for {
          N: w223 -> [_]
          tunnel: w217 -> [w235]
          tunnel: [w233] -> w222 mode=indexing
          i -> [w234]
          n91 = case shown="0, Default" w234 {
            tunnel: w235 -> [w241 w247 w253 w259 w265 w271 w277 w283 w289 w295 w301 w307 w313 w319 w325 w331 w337 w343 w349 w355]
            tunnel: [w236 w242 w248 w254 w260 w266 w272 w278 w284 w290 w296 w302 w308 w314 w320 w326 w332 w338 w344 w350] -> w233
            frame 0, Default {
              n92 = Unbundle By Name(w241) -> ("Eq1"=w239:timestamp)
              n93 = Get Date/Time In Seconds() -> (seconds since 1Jan1904=w240:timestamp)
              n94 = Get Date/Time String(seconds (now)=w239) -> (date string=w238:string)  [unwired: 2 in, 1 out]
              n95 = Get Date/Time String(seconds (now)=w240) -> (date string=w237:string)  [unwired: 2 in, 1 out]
              n96 = call "UTILITY Date String Days.vi"("First date"=w237, "Second date"=w238) -> ("Elapsed days"=w236:i32)  [unwired: 8 in, 1 out]
            }
            frame 1 {
              n97 = Unbundle By Name(w247) -> ("Eq2"=w243:timestamp)
              n98 = Get Date/Time In Seconds() -> (seconds since 1Jan1904=w246:timestamp)
              n99 = Get Date/Time String(seconds (now)=w243) -> (date string=w245:string)  [unwired: 2 in, 1 out]
              n100 = Get Date/Time String(seconds (now)=w246) -> (date string=w244:string)  [unwired: 2 in, 1 out]
              n101 = call "UTILITY Date String Days.vi"("First date"=w244, "Second date"=w245) -> ("Elapsed days"=w242:i32)  [unwired: 8 in, 1 out]
            }
            frame 2 {
              n102 = Unbundle By Name(w253) -> ("Eq3"=w249:timestamp)
              n103 = Get Date/Time In Seconds() -> (seconds since 1Jan1904=w252:timestamp)
              n104 = Get Date/Time String(seconds (now)=w249) -> (date string=w251:string)  [unwired: 2 in, 1 out]
              n105 = Get Date/Time String(seconds (now)=w252) -> (date string=w250:string)  [unwired: 2 in, 1 out]
              n106 = call "UTILITY Date String Days.vi"("First date"=w250, "Second date"=w251) -> ("Elapsed days"=w248:i32)  [unwired: 8 in, 1 out]
            }
            frame 3 {
              n107 = Unbundle By Name(w259) -> ("Eq4"=w255:timestamp)
              n108 = Get Date/Time In Seconds() -> (seconds since 1Jan1904=w258:timestamp)
              n109 = Get Date/Time String(seconds (now)=w255) -> (date string=w257:string)  [unwired: 2 in, 1 out]
              n110 = Get Date/Time String(seconds (now)=w258) -> (date string=w256:string)  [unwired: 2 in, 1 out]
              n111 = call "UTILITY Date String Days.vi"("First date"=w256, "Second date"=w257) -> ("Elapsed days"=w254:i32)  [unwired: 8 in, 1 out]
            }
            frame 4 {
              n112 = Unbundle By Name(w265) -> ("Eq5"=w261:timestamp)
              n113 = Get Date/Time In Seconds() -> (seconds since 1Jan1904=w264:timestamp)
              n114 = Get Date/Time String(seconds (now)=w261) -> (date string=w263:string)  [unwired: 2 in, 1 out]
              n115 = Get Date/Time String(seconds (now)=w264) -> (date string=w262:string)  [unwired: 2 in, 1 out]
              n116 = call "UTILITY Date String Days.vi"("First date"=w262, "Second date"=w263) -> ("Elapsed days"=w260:i32)  [unwired: 8 in, 1 out]
            }
            frame 5 {
              n117 = Unbundle By Name(w271) -> ("Eq6"=w267:timestamp)
              n118 = Get Date/Time In Seconds() -> (seconds since 1Jan1904=w270:timestamp)
              n119 = Get Date/Time String(seconds (now)=w267) -> (date string=w269:string)  [unwired: 2 in, 1 out]
              n120 = Get Date/Time String(seconds (now)=w270) -> (date string=w268:string)  [unwired: 2 in, 1 out]
              n121 = call "UTILITY Date String Days.vi"("First date"=w268, "Second date"=w269) -> ("Elapsed days"=w266:i32)  [unwired: 8 in, 1 out]
            }
            frame 6 {
              n122 = Unbundle By Name(w277) -> ("Eq7"=w273:timestamp)
              n123 = Get Date/Time In Seconds() -> (seconds since 1Jan1904=w276:timestamp)
              n124 = Get Date/Time String(seconds (now)=w273) -> (date string=w275:string)  [unwired: 2 in, 1 out]
              n125 = Get Date/Time String(seconds (now)=w276) -> (date string=w274:string)  [unwired: 2 in, 1 out]
              n126 = call "UTILITY Date String Days.vi"("First date"=w274, "Second date"=w275) -> ("Elapsed days"=w272:i32)  [unwired: 8 in, 1 out]
            }
            frame 7 {
              n127 = Unbundle By Name(w283) -> ("Eq8"=w279:timestamp)
              n128 = Get Date/Time In Seconds() -> (seconds since 1Jan1904=w282:timestamp)
              n129 = Get Date/Time String(seconds (now)=w279) -> (date string=w281:string)  [unwired: 2 in, 1 out]
              n130 = Get Date/Time String(seconds (now)=w282) -> (date string=w280:string)  [unwired: 2 in, 1 out]
              n131 = call "UTILITY Date String Days.vi"("First date"=w280, "Second date"=w281) -> ("Elapsed days"=w278:i32)  [unwired: 8 in, 1 out]
            }
            frame 8 {
              n132 = Unbundle By Name(w289) -> ("Eq9"=w285:timestamp)
              n133 = Get Date/Time In Seconds() -> (seconds since 1Jan1904=w288:timestamp)
              n134 = Get Date/Time String(seconds (now)=w285) -> (date string=w287:string)  [unwired: 2 in, 1 out]
              n135 = Get Date/Time String(seconds (now)=w288) -> (date string=w286:string)  [unwired: 2 in, 1 out]
              n136 = call "UTILITY Date String Days.vi"("First date"=w286, "Second date"=w287) -> ("Elapsed days"=w284:i32)  [unwired: 8 in, 1 out]
            }
            frame 9 {
              n137 = Unbundle By Name(w295) -> ("Eq10"=w291:timestamp)
              n138 = Get Date/Time In Seconds() -> (seconds since 1Jan1904=w294:timestamp)
              n139 = Get Date/Time String(seconds (now)=w291) -> (date string=w293:string)  [unwired: 2 in, 1 out]
              n140 = Get Date/Time String(seconds (now)=w294) -> (date string=w292:string)  [unwired: 2 in, 1 out]
              n141 = call "UTILITY Date String Days.vi"("First date"=w292, "Second date"=w293) -> ("Elapsed days"=w290:i32)  [unwired: 8 in, 1 out]
            }
            frame 10 {
              n142 = Unbundle By Name(w301) -> ("Eq11"=w297:timestamp)
              n143 = Get Date/Time In Seconds() -> (seconds since 1Jan1904=w300:timestamp)
              n144 = Get Date/Time String(seconds (now)=w297) -> (date string=w299:string)  [unwired: 2 in, 1 out]
              n145 = Get Date/Time String(seconds (now)=w300) -> (date string=w298:string)  [unwired: 2 in, 1 out]
              n146 = call "UTILITY Date String Days.vi"("First date"=w298, "Second date"=w299) -> ("Elapsed days"=w296:i32)  [unwired: 8 in, 1 out]
            }
            frame 11 {
              n147 = Unbundle By Name(w307) -> ("Eq12"=w303:timestamp)
              n148 = Get Date/Time In Seconds() -> (seconds since 1Jan1904=w306:timestamp)
              n149 = Get Date/Time String(seconds (now)=w303) -> (date string=w305:string)  [unwired: 2 in, 1 out]
              n150 = Get Date/Time String(seconds (now)=w306) -> (date string=w304:string)  [unwired: 2 in, 1 out]
              n151 = call "UTILITY Date String Days.vi"("First date"=w304, "Second date"=w305) -> ("Elapsed days"=w302:i32)  [unwired: 8 in, 1 out]
            }
            frame 12 {
              n152 = Unbundle By Name(w313) -> ("Eq13"=w309:timestamp)
              n153 = Get Date/Time In Seconds() -> (seconds since 1Jan1904=w312:timestamp)
              n154 = Get Date/Time String(seconds (now)=w309) -> (date string=w311:string)  [unwired: 2 in, 1 out]
              n155 = Get Date/Time String(seconds (now)=w312) -> (date string=w310:string)  [unwired: 2 in, 1 out]
              n156 = call "UTILITY Date String Days.vi"("First date"=w310, "Second date"=w311) -> ("Elapsed days"=w308:i32)  [unwired: 8 in, 1 out]
            }
            frame 13 {
              n157 = Unbundle By Name(w319) -> ("Eq14"=w315:timestamp)
              n158 = Get Date/Time In Seconds() -> (seconds since 1Jan1904=w318:timestamp)
              n159 = Get Date/Time String(seconds (now)=w315) -> (date string=w317:string)  [unwired: 2 in, 1 out]
              n160 = Get Date/Time String(seconds (now)=w318) -> (date string=w316:string)  [unwired: 2 in, 1 out]
              n161 = call "UTILITY Date String Days.vi"("First date"=w316, "Second date"=w317) -> ("Elapsed days"=w314:i32)  [unwired: 8 in, 1 out]
            }
            frame 14 {
              n162 = Unbundle By Name(w325) -> ("Eq15"=w321:timestamp)
              n163 = Get Date/Time In Seconds() -> (seconds since 1Jan1904=w324:timestamp)
              n164 = Get Date/Time String(seconds (now)=w321) -> (date string=w323:string)  [unwired: 2 in, 1 out]
              n165 = Get Date/Time String(seconds (now)=w324) -> (date string=w322:string)  [unwired: 2 in, 1 out]
              n166 = call "UTILITY Date String Days.vi"("First date"=w322, "Second date"=w323) -> ("Elapsed days"=w320:i32)  [unwired: 8 in, 1 out]
            }
            frame 15 {
              n167 = Unbundle By Name(w331) -> ("Eq16"=w327:timestamp)
              n168 = Get Date/Time In Seconds() -> (seconds since 1Jan1904=w330:timestamp)
              n169 = Get Date/Time String(seconds (now)=w327) -> (date string=w329:string)  [unwired: 2 in, 1 out]
              n170 = Get Date/Time String(seconds (now)=w330) -> (date string=w328:string)  [unwired: 2 in, 1 out]
              n171 = call "UTILITY Date String Days.vi"("First date"=w328, "Second date"=w329) -> ("Elapsed days"=w326:i32)  [unwired: 8 in, 1 out]
            }
            frame 16 {
              n172 = Unbundle By Name(w337) -> ("Eq17"=w333:timestamp)
              n173 = Get Date/Time In Seconds() -> (seconds since 1Jan1904=w336:timestamp)
              n174 = Get Date/Time String(seconds (now)=w333) -> (date string=w335:string)  [unwired: 2 in, 1 out]
              n175 = Get Date/Time String(seconds (now)=w336) -> (date string=w334:string)  [unwired: 2 in, 1 out]
              n176 = call "UTILITY Date String Days.vi"("First date"=w334, "Second date"=w335) -> ("Elapsed days"=w332:i32)  [unwired: 8 in, 1 out]
            }
            frame 17 {
              n177 = Unbundle By Name(w343) -> ("Eq18"=w339:timestamp)
              n178 = Get Date/Time In Seconds() -> (seconds since 1Jan1904=w342:timestamp)
              n179 = Get Date/Time String(seconds (now)=w339) -> (date string=w341:string)  [unwired: 2 in, 1 out]
              n180 = Get Date/Time String(seconds (now)=w342) -> (date string=w340:string)  [unwired: 2 in, 1 out]
              n181 = call "UTILITY Date String Days.vi"("First date"=w340, "Second date"=w341) -> ("Elapsed days"=w338:i32)  [unwired: 8 in, 1 out]
            }
            frame 18 {
              n182 = Unbundle By Name(w349) -> ("Eq19"=w345:timestamp)
              n183 = Get Date/Time In Seconds() -> (seconds since 1Jan1904=w348:timestamp)
              n184 = Get Date/Time String(seconds (now)=w345) -> (date string=w347:string)  [unwired: 2 in, 1 out]
              n185 = Get Date/Time String(seconds (now)=w348) -> (date string=w346:string)  [unwired: 2 in, 1 out]
              n186 = call "UTILITY Date String Days.vi"("First date"=w346, "Second date"=w347) -> ("Elapsed days"=w344:i32)  [unwired: 8 in, 1 out]
            }
            frame 19 {
              n187 = Unbundle By Name(w355) -> ("Eq20"=w351:timestamp)
              n188 = Get Date/Time In Seconds() -> (seconds since 1Jan1904=w354:timestamp)
              n189 = Get Date/Time String(seconds (now)=w351) -> (date string=w353:string)  [unwired: 2 in, 1 out]
              n190 = Get Date/Time String(seconds (now)=w354) -> (date string=w352:string)  [unwired: 2 in, 1 out]
              n191 = call "UTILITY Date String Days.vi"("First date"=w352, "Second date"=w353) -> ("Elapsed days"=w350:i32)  [unwired: 8 in, 1 out]
            }
          }
        }
        n192 = Array Max & Min(array=w222) -> (min value=w219:i32)  [unwired: 3 out]
        n193 = Number To Decimal String(number=w219) -> (decimal integer string=w218:string)  [unwired: 1 in]
        n194 = Less?(x=w219, y=30) -> (x < y?=w220:bool)
        n195 = case shown="True" w220 {
          tunnel: w218 -> [_ w232]
          tunnel: ["" w229] -> w216
          frame False {
          }
          frame True {
            n196 = Concatenate Strings("Componets will be out of calibration in " ("message"), w232, " Days" ("string")) -> (w229:string)
            n197 = One Button Dialog(message=w229) -> ()  [unwired: 1 in, 1 out]
          }
        }
        "concatenated string" <- w216
        n198 = call <vilib>:"Add State(s) to Queue__jki_lib_state_machine.vi"("State(s) in (\"\")"=w227) -> ("States Out"=w226:string)  [unwired: 14 in]
      }
      frame "Equipment Desc" {
        n199 = Unbundle By Name(w363) -> ("Total Array"=w356:string[][], "Equipment Description"=w361:T1)
        n200 = for {
          N: 20 -> [_]
          tunnel: w361 -> [w375]
          tunnel: string[] [] -> [w373]
          tunnel: [w372] -> w359 mode=indexing
          tunnel: [w371] -> w364
          tunnel: w365 -> [w371]
          i -> [w374]
          n201 = case shown="15" w374 {
            tunnel: w375 -> [w377 w379 w381 w383 w385 w387 w389 w391 w393 w395 w397 w399 w401 w403 w405 w407 w409 w410 w413 w415]
            tunnel: [w376 w378 w380 w382 w384 w386 w388 w390 w392 w394 w396 w398 w400 w402 w404 w406 w408 w411 w412 w414] -> w370
            frame 0, Default {
              n202 = Unbundle By Name(w377) -> ("Eq 1"=w376:string)
            }
            frame 1 {
              n203 = Unbundle By Name(w379) -> ("Eq 2"=w378:string)
            }
            frame 2 {
              n204 = Unbundle By Name(w381) -> ("Eq 3"=w380:string)
            }
            frame 3 {
              n205 = Unbundle By Name(w383) -> ("Eq 4"=w382:string)
            }
            frame 4 {
              n206 = Unbundle By Name(w385) -> ("Eq 5"=w384:string)
            }
            frame 5 {
              n207 = Unbundle By Name(w387) -> ("Eq 6"=w386:string)
            }
            frame 6 {
              n208 = Unbundle By Name(w389) -> ("Eq 7"=w388:string)
            }
            frame 7 {
              n209 = Unbundle By Name(w391) -> ("Eq 8"=w390:string)
            }
            frame 8 {
              n210 = Unbundle By Name(w393) -> ("Eq 9"=w392:string)
            }
            frame 9 {
              n211 = Unbundle By Name(w395) -> ("Eq 10"=w394:string)
            }
            frame 10 {
              n212 = Unbundle By Name(w397) -> ("Eq 11"=w396:string)
            }
            frame 11 {
              n213 = Unbundle By Name(w399) -> ("Eq 12"=w398:string)
            }
            frame 12 {
              n214 = Unbundle By Name(w401) -> ("Eq 13"=w400:string)
            }
            frame 13 {
              n215 = Unbundle By Name(w403) -> ("Eq 14"=w402:string)
            }
            frame 14 {
              n216 = Unbundle By Name(w405) -> ("Eq 15"=w404:string)
            }
            frame 15 {
              n217 = Unbundle By Name(w407) -> ("Eq 16"=w406:string)
            }
            frame 16 {
              n218 = Unbundle By Name(w409) -> ("Eq 17"=w408:string)
            }
            frame 17 {
              n219 = Unbundle By Name(w410) -> ("Eq 18"=w411:string)
            }
            frame 18 {
              n220 = Unbundle By Name(w413) -> ("Eq 19"=w412:string)
            }
            frame 19 {
              n221 = Unbundle By Name(w415) -> ("Eq 20"=w414:string)
            }
          }
          n222 = Build Array (concatenate)(w373, w370) -> (w372:string[])
        }
        n223 = call "UTILITY Array Get 1D String Column From 2D.vi"("2D Array Data"=w359, "column index"=0) -> ("Column Data"=w357:string[])  [unwired: 13 in]
        n224 = Build Array (concatenate)(w356, w357) -> (w360:string[][])
        n225 = Bundle By Name(cluster=w363, "Total Array"=w360) -> (w362:T8)
        n226 = call <vilib>:"Add State(s) to Queue__jki_lib_state_machine.vi"("State(s) in (\"\")"=w369) -> ("States Out"=w368:string)  [unwired: 14 in]
      }
      frame "Manufacturer" {
        n227 = Unbundle By Name(w423) -> ("Manufacturer"=w421:T1, "Total Array"=w420:string[][])
        n228 = for {
          N: 20 -> [_]
          tunnel: w421 -> [w435]
          tunnel: string[] [] -> [w433]
          tunnel: [w432] -> w418 mode=indexing
          tunnel: [w431] -> w424
          tunnel: w425 -> [w431]
          i -> [w434]
          n229 = case shown="15" w434 {
            tunnel: w435 -> [w437 w439 w441 w443 w445 w447 w449 w451 w453 w455 w457 w459 w461 w463 w465 w467 w469 w470 w473 w475]
            tunnel: [w436 w438 w440 w442 w444 w446 w448 w450 w452 w454 w456 w458 w460 w462 w464 w466 w468 w471 w472 w474] -> w430
            frame 0, Default {
              n230 = Unbundle By Name(w437) -> ("Eq 1"=w436:string)
            }
            frame 1 {
              n231 = Unbundle By Name(w439) -> ("Eq 2"=w438:string)
            }
            frame 2 {
              n232 = Unbundle By Name(w441) -> ("Eq 3"=w440:string)
            }
            frame 3 {
              n233 = Unbundle By Name(w443) -> ("Eq 4"=w442:string)
            }
            frame 4 {
              n234 = Unbundle By Name(w445) -> ("Eq 5"=w444:string)
            }
            frame 5 {
              n235 = Unbundle By Name(w447) -> ("Eq 6"=w446:string)
            }
            frame 6 {
              n236 = Unbundle By Name(w449) -> ("Eq 7"=w448:string)
            }
            frame 7 {
              n237 = Unbundle By Name(w451) -> ("Eq 8"=w450:string)
            }
            frame 8 {
              n238 = Unbundle By Name(w453) -> ("Eq 9"=w452:string)
            }
            frame 9 {
              n239 = Unbundle By Name(w455) -> ("Eq 10"=w454:string)
            }
            frame 10 {
              n240 = Unbundle By Name(w457) -> ("Eq 11"=w456:string)
            }
            frame 11 {
              n241 = Unbundle By Name(w459) -> ("Eq 12"=w458:string)
            }
            frame 12 {
              n242 = Unbundle By Name(w461) -> ("Eq 13"=w460:string)
            }
            frame 13 {
              n243 = Unbundle By Name(w463) -> ("Eq 14"=w462:string)
            }
            frame 14 {
              n244 = Unbundle By Name(w465) -> ("Eq 15"=w464:string)
            }
            frame 15 {
              n245 = Unbundle By Name(w467) -> ("Eq 16"=w466:string)
            }
            frame 16 {
              n246 = Unbundle By Name(w469) -> ("Eq 17"=w468:string)
            }
            frame 17 {
              n247 = Unbundle By Name(w470) -> ("Eq 18"=w471:string)
            }
            frame 18 {
              n248 = Unbundle By Name(w473) -> ("Eq 19"=w472:string)
            }
            frame 19 {
              n249 = Unbundle By Name(w475) -> ("Eq 20"=w474:string)
            }
          }
          n250 = Build Array (concatenate)(w433, w430) -> (w432:string[])
        }
        n251 = call "UTILITY Array Get 1D String Column From 2D.vi"("2D Array Data"=w418, "column index"=0) -> ("Column Data"=w416:string[])  [unwired: 13 in]
        n252 = Build Array (concatenate)(w420, w416) -> (w419:string[][])
        n253 = Bundle By Name(cluster=w423, "Total Array"=w419) -> (w422:T8)
        n254 = call <vilib>:"Add State(s) to Queue__jki_lib_state_machine.vi"("State(s) in (\"\")"=w429) -> ("States Out"=w428:string)  [unwired: 14 in]
      }
      frame "Model Number" {
        n255 = Unbundle By Name(w483) -> ("Model Number"=w481:T1, "Total Array"=w480:string[][])
        n256 = for {
          N: 20 -> [_]
          tunnel: w481 -> [w495]
          tunnel: string[] [] -> [w493]
          tunnel: [w492] -> w478 mode=indexing
          tunnel: [w491] -> w484
          tunnel: w485 -> [w491]
          i -> [w494]
          n257 = case shown="15" w494 {
            tunnel: w495 -> [w497 w499 w501 w503 w505 w507 w509 w511 w513 w515 w517 w519 w521 w523 w525 w527 w529 w530 w533 w535]
            tunnel: [w496 w498 w500 w502 w504 w506 w508 w510 w512 w514 w516 w518 w520 w522 w524 w526 w528 w531 w532 w534] -> w490
            frame 0, Default {
              n258 = Unbundle By Name(w497) -> ("Eq 1"=w496:string)
            }
            frame 1 {
              n259 = Unbundle By Name(w499) -> ("Eq 2"=w498:string)
            }
            frame 2 {
              n260 = Unbundle By Name(w501) -> ("Eq 3"=w500:string)
            }
            frame 3 {
              n261 = Unbundle By Name(w503) -> ("Eq 4"=w502:string)
            }
            frame 4 {
              n262 = Unbundle By Name(w505) -> ("Eq 5"=w504:string)
            }
            frame 5 {
              n263 = Unbundle By Name(w507) -> ("Eq 6"=w506:string)
            }
            frame 6 {
              n264 = Unbundle By Name(w509) -> ("Eq 7"=w508:string)
            }
            frame 7 {
              n265 = Unbundle By Name(w511) -> ("Eq 8"=w510:string)
            }
            frame 8 {
              n266 = Unbundle By Name(w513) -> ("Eq 9"=w512:string)
            }
            frame 9 {
              n267 = Unbundle By Name(w515) -> ("Eq 10"=w514:string)
            }
            frame 10 {
              n268 = Unbundle By Name(w517) -> ("Eq 11"=w516:string)
            }
            frame 11 {
              n269 = Unbundle By Name(w519) -> ("Eq 12"=w518:string)
            }
            frame 12 {
              n270 = Unbundle By Name(w521) -> ("Eq 13"=w520:string)
            }
            frame 13 {
              n271 = Unbundle By Name(w523) -> ("Eq 14"=w522:string)
            }
            frame 14 {
              n272 = Unbundle By Name(w525) -> ("Eq 15"=w524:string)
            }
            frame 15 {
              n273 = Unbundle By Name(w527) -> ("Eq 16"=w526:string)
            }
            frame 16 {
              n274 = Unbundle By Name(w529) -> ("Eq 17"=w528:string)
            }
            frame 17 {
              n275 = Unbundle By Name(w530) -> ("Eq 18"=w531:string)
            }
            frame 18 {
              n276 = Unbundle By Name(w533) -> ("Eq 19"=w532:string)
            }
            frame 19 {
              n277 = Unbundle By Name(w535) -> ("Eq 20"=w534:string)
            }
          }
          n278 = Build Array (concatenate)(w493, w490) -> (w492:string[])
        }
        n279 = call "UTILITY Array Get 1D String Column From 2D.vi"("2D Array Data"=w478, "column index"=0) -> ("Column Data"=w476:string[])  [unwired: 13 in]
        n280 = Build Array (concatenate)(w480, w476) -> (w479:string[][])
        n281 = Bundle By Name(cluster=w483, "Total Array"=w479) -> (w482:T8)
        n282 = call <vilib>:"Add State(s) to Queue__jki_lib_state_machine.vi"("State(s) in (\"\")"=w489) -> ("States Out"=w488:string)  [unwired: 14 in]
      }
      frame "Write Calibration ID" {
        n283 = Unbundle By Name(w543) -> ("Calibration ID"=w541:T1, "Total Array"=w540:string[][])
        n284 = for {
          N: 20 -> [_]
          tunnel: w541 -> [w555]
          tunnel: string[] [] -> [w553]
          tunnel: [w552] -> w538 mode=indexing
          tunnel: [w551] -> w544
          tunnel: w545 -> [w551]
          i -> [w554]
          n285 = case shown="15" w554 {
            tunnel: w555 -> [w557 w559 w561 w563 w565 w567 w569 w571 w573 w575 w577 w579 w581 w583 w585 w587 w589 w590 w593 w595]
            tunnel: [w556 w558 w560 w562 w564 w566 w568 w570 w572 w574 w576 w578 w580 w582 w584 w586 w588 w591 w592 w594] -> w550
            frame 0, Default {
              n286 = Unbundle By Name(w557) -> ("Eq 1"=w556:string)
            }
            frame 1 {
              n287 = Unbundle By Name(w559) -> ("Eq 2"=w558:string)
            }
            frame 2 {
              n288 = Unbundle By Name(w561) -> ("Eq 3"=w560:string)
            }
            frame 3 {
              n289 = Unbundle By Name(w563) -> ("Eq 4"=w562:string)
            }
            frame 4 {
              n290 = Unbundle By Name(w565) -> ("Eq 5"=w564:string)
            }
            frame 5 {
              n291 = Unbundle By Name(w567) -> ("Eq 6"=w566:string)
            }
            frame 6 {
              n292 = Unbundle By Name(w569) -> ("Eq 7"=w568:string)
            }
            frame 7 {
              n293 = Unbundle By Name(w571) -> ("Eq 8"=w570:string)
            }
            frame 8 {
              n294 = Unbundle By Name(w573) -> ("Eq 9"=w572:string)
            }
            frame 9 {
              n295 = Unbundle By Name(w575) -> ("Eq 10"=w574:string)
            }
            frame 10 {
              n296 = Unbundle By Name(w577) -> ("Eq 11"=w576:string)
            }
            frame 11 {
              n297 = Unbundle By Name(w579) -> ("Eq 12"=w578:string)
            }
            frame 12 {
              n298 = Unbundle By Name(w581) -> ("Eq 13"=w580:string)
            }
            frame 13 {
              n299 = Unbundle By Name(w583) -> ("Eq 14"=w582:string)
            }
            frame 14 {
              n300 = Unbundle By Name(w585) -> ("Eq 15"=w584:string)
            }
            frame 15 {
              n301 = Unbundle By Name(w587) -> ("Eq 16"=w586:string)
            }
            frame 16 {
              n302 = Unbundle By Name(w589) -> ("Eq 17"=w588:string)
            }
            frame 17 {
              n303 = Unbundle By Name(w590) -> ("Eq 18"=w591:string)
            }
            frame 18 {
              n304 = Unbundle By Name(w593) -> ("Eq 19"=w592:string)
            }
            frame 19 {
              n305 = Unbundle By Name(w595) -> ("Eq 20"=w594:string)
            }
          }
          n306 = Build Array (concatenate)(w553, w550) -> (w552:string[])
        }
        n307 = call "UTILITY Array Get 1D String Column From 2D.vi"("2D Array Data"=w538, "column index"=0) -> ("Column Data"=w536:string[])  [unwired: 13 in]
        n308 = Build Array (concatenate)(w540, w536) -> (w539:string[][])
        n309 = Bundle By Name(cluster=w543, "Total Array"=w539) -> (w542:T8)
        n310 = call <vilib>:"Add State(s) to Queue__jki_lib_state_machine.vi"("State(s) in (\"\")"=w549) -> ("States Out"=w548:string)  [unwired: 14 in]
      }
      frame "Write Calibration SN" {
        n311 = Unbundle By Name(w603) -> ("Serial Number"=w601:T2, "Total Array"=w600:string[][])
        n312 = for {
          N: 20 -> [_]
          tunnel: w601 -> [w615]
          tunnel: string[] [] -> [w613]
          tunnel: [w612] -> w598 mode=indexing
          tunnel: [w611] -> w604
          tunnel: w605 -> [w611]
          i -> [w614]
          n313 = case shown="15" w614 {
            tunnel: w615 -> [w617 w619 w621 w623 w625 w627 w629 w631 w633 w635 w637 w639 w641 w643 w645 w647 w649 w651 w653 w655]
            tunnel: [w616 w618 w620 w622 w624 w626 w628 w630 w632 w634 w636 w638 w640 w642 w644 w646 w648 w650 w652 w654] -> w610
            frame 0, Default {
              n314 = Unbundle By Name(w617) -> ("Eq 1"=w616:string)
            }
            frame 1 {
              n315 = Unbundle By Name(w619) -> ("Eq 2"=w618:string)
            }
            frame 2 {
              n316 = Unbundle By Name(w621) -> ("Eq 3"=w620:string)
            }
            frame 3 {
              n317 = Unbundle By Name(w623) -> ("Eq 4"=w622:string)
            }
            frame 4 {
              n318 = Unbundle By Name(w625) -> ("Eq 5"=w624:string)
            }
            frame 5 {
              n319 = Unbundle By Name(w627) -> ("Eq 6"=w626:string)
            }
            frame 6 {
              n320 = Unbundle By Name(w629) -> ("Eq 7"=w628:string)
            }
            frame 7 {
              n321 = Unbundle By Name(w631) -> ("Eq 8"=w630:string)
            }
            frame 8 {
              n322 = Unbundle By Name(w633) -> ("Eq 9"=w632:string)
            }
            frame 9 {
              n323 = Unbundle By Name(w635) -> ("Eq 10"=w634:string)
            }
            frame 10 {
              n324 = Unbundle By Name(w637) -> ("Eq 11"=w636:string)
            }
            frame 11 {
              n325 = Unbundle By Name(w639) -> ("Eq 12"=w638:string)
            }
            frame 12 {
              n326 = Unbundle By Name(w641) -> ("Eq 13"=w640:string)
            }
            frame 13 {
              n327 = Unbundle By Name(w643) -> ("Eq 14"=w642:string)
            }
            frame 14 {
              n328 = Unbundle By Name(w645) -> ("Eq 15"=w644:string)
            }
            frame 15 {
              n329 = Unbundle By Name(w647) -> ("Eq 16"=w646:string)
            }
            frame 16 {
              n330 = Unbundle By Name(w649) -> ("Eq 17"=w648:string)
            }
            frame 17 {
              n331 = Unbundle By Name(w651) -> ("Eq 18"=w650:string)
            }
            frame 18 {
              n332 = Unbundle By Name(w653) -> ("Eq 19"=w652:string)
            }
            frame 19 {
              n333 = Unbundle By Name(w655) -> ("Eq 20"=w654:string)
            }
          }
          n334 = Build Array (concatenate)(w613, w610) -> (w612:string[])
        }
        n335 = call "UTILITY Array Get 1D String Column From 2D.vi"("2D Array Data"=w598, "column index"=0) -> ("Column Data"=w596:string[])  [unwired: 13 in]
        "snta" <- w596
        n336 = Build Array (concatenate)(w600, w596) -> (w599:string[][])
        n337 = Bundle By Name(cluster=w603, "Total Array"=w599) -> (w602:T8)
        n338 = call <vilib>:"Add State(s) to Queue__jki_lib_state_machine.vi"("State(s) in (\"\")"=w609) -> ("States Out"=w608:string)  [unwired: 14 in]
      }
      frame "Last Calibration" {
        n339 = Unbundle By Name(w662) -> ("Last Calibrated"=w663:T3, "Total Array"=w658:string[][])
        n340 = for {
          N: 20 -> [_]
          tunnel: w663 -> [w677]
          tunnel: string[] [] -> [w675]
          tunnel: [w674] -> w660 mode=indexing
          tunnel: [w670] -> w664
          tunnel: w665 -> [w670]
          i -> [w676]
          n341 = case shown="0, Default" w676 {
            tunnel: w677 -> [w680 w683 w686 w689 w692 w695 w698 w701 w704 w707 w710 w713 w716 w719 w722 w725 w728 w731 w733 w737]
            tunnel: [w678 w681 w684 w687 w690 w693 w696 w699 w702 w705 w708 w711 w714 w717 w720 w723 w726 w729 w734 w735] -> w673
            frame 0, Default {
              n342 = Unbundle By Name(w680) -> ("Eq1"=w679:timestamp)
              n343 = Format Date/Time String(seconds (now)=w679) -> (date/time string=w678:string)  [unwired: 2 in]
            }
            frame 1 {
              n344 = Unbundle By Name(w683) -> ("Eq2"=w682:timestamp)
              n345 = Format Date/Time String(seconds (now)=w682) -> (date/time string=w681:string)  [unwired: 2 in]
            }
            frame 2 {
              n346 = Unbundle By Name(w686) -> ("Eq3"=w685:timestamp)
              n347 = Format Date/Time String(seconds (now)=w685) -> (date/time string=w684:string)  [unwired: 2 in]
            }
            frame 3 {
              n348 = Unbundle By Name(w689) -> ("Eq4"=w688:timestamp)
              n349 = Format Date/Time String(seconds (now)=w688) -> (date/time string=w687:string)  [unwired: 2 in]
            }
            frame 4 {
              n350 = Unbundle By Name(w692) -> ("Eq5"=w691:timestamp)
              n351 = Format Date/Time String(seconds (now)=w691) -> (date/time string=w690:string)  [unwired: 2 in]
            }
            frame 5 {
              n352 = Unbundle By Name(w695) -> ("Eq6"=w694:timestamp)
              n353 = Format Date/Time String(seconds (now)=w694) -> (date/time string=w693:string)  [unwired: 2 in]
            }
            frame 6 {
              n354 = Unbundle By Name(w698) -> ("Eq7"=w697:timestamp)
              n355 = Format Date/Time String(seconds (now)=w697) -> (date/time string=w696:string)  [unwired: 2 in]
            }
            frame 7 {
              n356 = Unbundle By Name(w701) -> ("Eq8"=w700:timestamp)
              n357 = Format Date/Time String(seconds (now)=w700) -> (date/time string=w699:string)  [unwired: 2 in]
            }
            frame 8 {
              n358 = Unbundle By Name(w704) -> ("Eq9"=w703:timestamp)
              n359 = Format Date/Time String(seconds (now)=w703) -> (date/time string=w702:string)  [unwired: 2 in]
            }
            frame 9 {
              n360 = Unbundle By Name(w707) -> ("Eq10"=w706:timestamp)
              n361 = Format Date/Time String(seconds (now)=w706) -> (date/time string=w705:string)  [unwired: 2 in]
            }
            frame 10 {
              n362 = Unbundle By Name(w710) -> ("Eq11"=w709:timestamp)
              n363 = Format Date/Time String(seconds (now)=w709) -> (date/time string=w708:string)  [unwired: 2 in]
            }
            frame 11 {
              n364 = Unbundle By Name(w713) -> ("Eq12"=w712:timestamp)
              n365 = Format Date/Time String(seconds (now)=w712) -> (date/time string=w711:string)  [unwired: 2 in]
            }
            frame 12 {
              n366 = Unbundle By Name(w716) -> ("Eq13"=w715:timestamp)
              n367 = Format Date/Time String(seconds (now)=w715) -> (date/time string=w714:string)  [unwired: 2 in]
            }
            frame 13 {
              n368 = Unbundle By Name(w719) -> ("Eq14"=w718:timestamp)
              n369 = Format Date/Time String(seconds (now)=w718) -> (date/time string=w717:string)  [unwired: 2 in]
            }
            frame 14 {
              n370 = Unbundle By Name(w722) -> ("Eq15"=w721:timestamp)
              n371 = Format Date/Time String(seconds (now)=w721) -> (date/time string=w720:string)  [unwired: 2 in]
            }
            frame 15 {
              n372 = Unbundle By Name(w725) -> ("Eq16"=w724:timestamp)
              n373 = Format Date/Time String(seconds (now)=w724) -> (date/time string=w723:string)  [unwired: 2 in]
            }
            frame 16 {
              n374 = Unbundle By Name(w728) -> ("Eq17"=w727:timestamp)
              n375 = Format Date/Time String(seconds (now)=w727) -> (date/time string=w726:string)  [unwired: 2 in]
            }
            frame 17 {
              n376 = Unbundle By Name(w731) -> ("Eq18"=w730:timestamp)
              n377 = Format Date/Time String(seconds (now)=w730) -> (date/time string=w729:string)  [unwired: 2 in]
            }
            frame 18 {
              n378 = Unbundle By Name(w733) -> ("Eq19"=w732:timestamp)
              n379 = Format Date/Time String(seconds (now)=w732) -> (date/time string=w734:string)  [unwired: 2 in]
            }
            frame 19 {
              n380 = Unbundle By Name(w737) -> ("Eq20"=w736:timestamp)
              n381 = Format Date/Time String(seconds (now)=w736) -> (date/time string=w735:string)  [unwired: 2 in]
            }
          }
          n382 = call <vilib>:"Space Constant.vi"() -> ("String"=w671:string)
          n383 = Match Pattern(string=w673, regular expression=w671) -> (before substring=w672:string)  [unwired: 1 in, 3 out]
          n384 = Build Array (concatenate)(w675, w672) -> (w674:string[])
        }
        n385 = call "UTILITY Array Get 1D String Column From 2D.vi"("2D Array Data"=w660, "column index"=0) -> ("Column Data"=w657:string[])  [unwired: 13 in]
        n386 = Build Array (concatenate)(w658, w657) -> (w656:string[][])
        n387 = Bundle By Name(cluster=w662, "Total Array"=w656) -> (w661:T8)
        n388 = call <vilib>:"Add State(s) to Queue__jki_lib_state_machine.vi"("State(s) in (\"\")"=w669) -> ("States Out"=w668:string)  [unwired: 14 in]
      }
      frame "Write Calibration Date" {
        n389 = Unbundle By Name(w744) -> ("Calibration Due"=w745:T3, "Total Array"=w740:string[][])
        n390 = for {
          N: 20 -> [_]
          tunnel: w745 -> [w759]
          tunnel: string[] [] -> [w757]
          tunnel: [w756] -> w742 mode=indexing
          tunnel: [w752] -> w746
          tunnel: w747 -> [w752]
          i -> [w758]
          n391 = case shown="15" w758 {
            tunnel: w759 -> [w762 w765 w768 w771 w774 w777 w780 w783 w786 w789 w792 w795 w798 w801 w804 w807 w810 w813 w815 w819]
            tunnel: [w760 w763 w766 w769 w772 w775 w778 w781 w784 w787 w790 w793 w796 w799 w802 w805 w808 w811 w816 w817] -> w755
            frame 0, Default {
              n392 = Unbundle By Name(w762) -> ("Eq1"=w761:timestamp)
              n393 = Format Date/Time String(seconds (now)=w761) -> (date/time string=w760:string)  [unwired: 2 in]
            }
            frame 1 {
              n394 = Unbundle By Name(w765) -> ("Eq2"=w764:timestamp)
              n395 = Format Date/Time String(seconds (now)=w764) -> (date/time string=w763:string)  [unwired: 2 in]
            }
            frame 2 {
              n396 = Unbundle By Name(w768) -> ("Eq3"=w767:timestamp)
              n397 = Format Date/Time String(seconds (now)=w767) -> (date/time string=w766:string)  [unwired: 2 in]
            }
            frame 3 {
              n398 = Unbundle By Name(w771) -> ("Eq4"=w770:timestamp)
              n399 = Format Date/Time String(seconds (now)=w770) -> (date/time string=w769:string)  [unwired: 2 in]
            }
            frame 4 {
              n400 = Unbundle By Name(w774) -> ("Eq5"=w773:timestamp)
              n401 = Format Date/Time String(seconds (now)=w773) -> (date/time string=w772:string)  [unwired: 2 in]
            }
            frame 5 {
              n402 = Unbundle By Name(w777) -> ("Eq6"=w776:timestamp)
              n403 = Format Date/Time String(seconds (now)=w776) -> (date/time string=w775:string)  [unwired: 2 in]
            }
            frame 6 {
              n404 = Unbundle By Name(w780) -> ("Eq7"=w779:timestamp)
              n405 = Format Date/Time String(seconds (now)=w779) -> (date/time string=w778:string)  [unwired: 2 in]
            }
            frame 7 {
              n406 = Unbundle By Name(w783) -> ("Eq8"=w782:timestamp)
              n407 = Format Date/Time String(seconds (now)=w782) -> (date/time string=w781:string)  [unwired: 2 in]
            }
            frame 8 {
              n408 = Unbundle By Name(w786) -> ("Eq9"=w785:timestamp)
              n409 = Format Date/Time String(seconds (now)=w785) -> (date/time string=w784:string)  [unwired: 2 in]
            }
            frame 9 {
              n410 = Unbundle By Name(w789) -> ("Eq10"=w788:timestamp)
              n411 = Format Date/Time String(seconds (now)=w788) -> (date/time string=w787:string)  [unwired: 2 in]
            }
            frame 10 {
              n412 = Unbundle By Name(w792) -> ("Eq11"=w791:timestamp)
              n413 = Format Date/Time String(seconds (now)=w791) -> (date/time string=w790:string)  [unwired: 2 in]
            }
            frame 11 {
              n414 = Unbundle By Name(w795) -> ("Eq12"=w794:timestamp)
              n415 = Format Date/Time String(seconds (now)=w794) -> (date/time string=w793:string)  [unwired: 2 in]
            }
            frame 12 {
              n416 = Unbundle By Name(w798) -> ("Eq13"=w797:timestamp)
              n417 = Format Date/Time String(seconds (now)=w797) -> (date/time string=w796:string)  [unwired: 2 in]
            }
            frame 13 {
              n418 = Unbundle By Name(w801) -> ("Eq14"=w800:timestamp)
              n419 = Format Date/Time String(seconds (now)=w800) -> (date/time string=w799:string)  [unwired: 2 in]
            }
            frame 14 {
              n420 = Unbundle By Name(w804) -> ("Eq15"=w803:timestamp)
              n421 = Format Date/Time String(seconds (now)=w803) -> (date/time string=w802:string)  [unwired: 2 in]
            }
            frame 15 {
              n422 = Unbundle By Name(w807) -> ("Eq16"=w806:timestamp)
              n423 = Format Date/Time String(seconds (now)=w806) -> (date/time string=w805:string)  [unwired: 2 in]
            }
            frame 16 {
              n424 = Unbundle By Name(w810) -> ("Eq17"=w809:timestamp)
              n425 = Format Date/Time String(seconds (now)=w809) -> (date/time string=w808:string)  [unwired: 2 in]
            }
            frame 17 {
              n426 = Unbundle By Name(w813) -> ("Eq18"=w812:timestamp)
              n427 = Format Date/Time String(seconds (now)=w812) -> (date/time string=w811:string)  [unwired: 2 in]
            }
            frame 18 {
              n428 = Unbundle By Name(w815) -> ("Eq19"=w814:timestamp)
              n429 = Format Date/Time String(seconds (now)=w814) -> (date/time string=w816:string)  [unwired: 2 in]
            }
            frame 19 {
              n430 = Unbundle By Name(w819) -> ("Eq20"=w818:timestamp)
              n431 = Format Date/Time String(seconds (now)=w818) -> (date/time string=w817:string)  [unwired: 2 in]
            }
          }
          n432 = call <vilib>:"Space Constant.vi"() -> ("String"=w753:string)
          n433 = Match Pattern(string=w755, regular expression=w753) -> (before substring=w754:string)  [unwired: 1 in, 3 out]
          n434 = Build Array (concatenate)(w757, w754) -> (w756:string[])
        }
        n435 = call "UTILITY Array Get 1D String Column From 2D.vi"("2D Array Data"=w742, "column index"=0) -> ("Column Data"=w739:string[])  [unwired: 13 in]
        n436 = Build Array (concatenate)(w740, w739) -> (w738:string[][])
        n437 = Bundle By Name(cluster=w744, "Total Array"=w738) -> (w743:T8)
        n438 = call <vilib>:"Add State(s) to Queue__jki_lib_state_machine.vi"("State(s) in (\"\")"=w751) -> ("States Out"=w750:string)  [unwired: 14 in]
      }
      frame "Write to File" {
        n439 = Unbundle By Name(w828) -> ("Calibration File Path"=w827:path, "Total Array"=w824:string[][])
        n440 = Transpose 2D Array(2D array=w824) -> (transposed array=w820:string[][])
        n441 = Build Array (concatenate)(string[] ["Equipment Description", "Manufacturer", "Model Number", "Calibration ID", "Serial Number", "Last Calibrated", "Calibration Due"], w820) -> (w822:string[][])
        n442 = call "UTILITY Delete Empty String Cells 2D.vi"("Array with Empty Cells"=w822) -> ("Array w/o Empty Cells"=→"Calibration Data":string[][])  [unwired: 10 in]
        n443 = call <vilib>:"Add State(s) to Queue__jki_lib_state_machine.vi"("State(s) in (\"\")"=w830) -> ("States Out"=w829:string)  [unwired: 14 in]
        n444 = call-poly <vilib>:"Write Delimited Spreadsheet.vi"("file path (dialog if empty)"=w827, "2D data"=w820, "delimiter (\\t)"="," ("delimiter (\\t)")) -> ()  [unwired: 11 in, 2 out]
      }
    }
  }
  "error out" <- w2
